vi "OBJ_MAIN.vi"() -> ()   [LabVIEW 2020]
uses:
  OBJ/MAIN/OBJ_header_data_display.ctl
  OBJ/ini/typedef/OBJ_all_config_info.ctl
  OBJ/ini/typedef/OBJ_main_ini_file.ctl
  OBJ/queues/typedef/OBJ_queue_refnums.ctl
  OBJ/queues/typedef/OBJ_MAIN_queue_element.ctl
  OBJ/MAIN/OBJ_MAIN_sequence_state.ctl
  OBJ/queues/typedef/OBJ_SCANNER_queue_element.ctl
  OBJ/SCANNER/OBJ_SCANNER_sequence_state.ctl
  OBJ/queues/typedef/OBJ_MD_queue_element.ctl
  OBJ/MEASURING_DEVICE/OBJ_MD_sequence_state.ctl
  OBJ/queues/typedef/OBJ_GUI_TIMER_queue_element.ctl
  OBJ/GUI_TIMER/OBJ_GUI_TIMER_sequence_state.ctl
  OBJ/FGV/error_buffer/FGV_OBJ_error_buffer.ctl
  OBJ/FGV/SQL_connection/FGV_OBJ_SQL_connection.ctl
  OBJ/FGV/login/FGV_OBJ_login.ctl
  OBJ/FGV/login/OBJ_login_refnums.ctl
  OBJ/FGV/test_button/FGV_OBJ_test_button.ctl
  OBJ/FGV/OBJ_records_display/FGV_OBJ_records_display.ctl
  OBJ/FGV/OBJ_status_display/FGV_OBJ_status_display.ctl
  OBJ/FGV/OBJ_records_display/OBJ_references.ctl
  OBJ/FGV/tristate_indicator_OBJ_test/FGV_tristate_indicator_OBJ_test.ctl
  OBJ/FGV/OBJ_history_display/FGV_OBJ_history_display.ctl
  OBJ/MAIN/OBJ_thread.ctl
  OBJ/FGV/part_number/control_part_number.ctl
  _misc/AULocalize/SubVIs/RegisterVI.vi
  <vilib>/Instr/_visa.llb/VISA Configure Serial Port (Instr).vi
  _misc/AULocalize/SubVIs/Get Localized Phrase Compact Interface 0D.vi
panel:
  out "tooling_name":string caption="Reference:"
  out "app_title":string caption="A603 - OBJ Position"
  in  "professional_timeout_reset_generator":bool
  in  "USER_login_logout":bool
  out "SQL_connections_indicator_global":bool=TRUE caption="SQL Connection Status:"
  out "ERROR_indicator_global":bool caption="Application Status:"
  out "current_access_level":i32=10 caption="Access level:"
  out "current_username":string="jlonga" caption="Logged in as:"
  in  "main_tab":enum32{"OBJ Test", "Errors"}(tab)
  out "input_header":string caption="INPUT"
  in  "OBJ_clear_history":bool
  in  "OBJ_clear_test_data":bool
  out "operator_message":string
  out "test_tristate_indicator":bool
  in  "OBJ_perform_test":bool
  out "OBJ_status":string
  in  "OBJ_gear_serial":string caption="Gear Serial:"
  out "OBJ_header_data_display":T1
  out "gear_info_summary_header":string caption="GEAR INFO SUMMARY"
  out "gear_serial_display":string
  out "OBJ_records":i32(listbox)=-1
  in  "OBJ_history":i32(listbox)=-1
  out "measurement_history_header":string caption="MEASUREMENT HISTORY"
  in  "ERROR_records":i32(listbox)
  in  "ERROR_clear":bool
  out "ERROR_indicator_tab":bool
  in  "STOP":bool
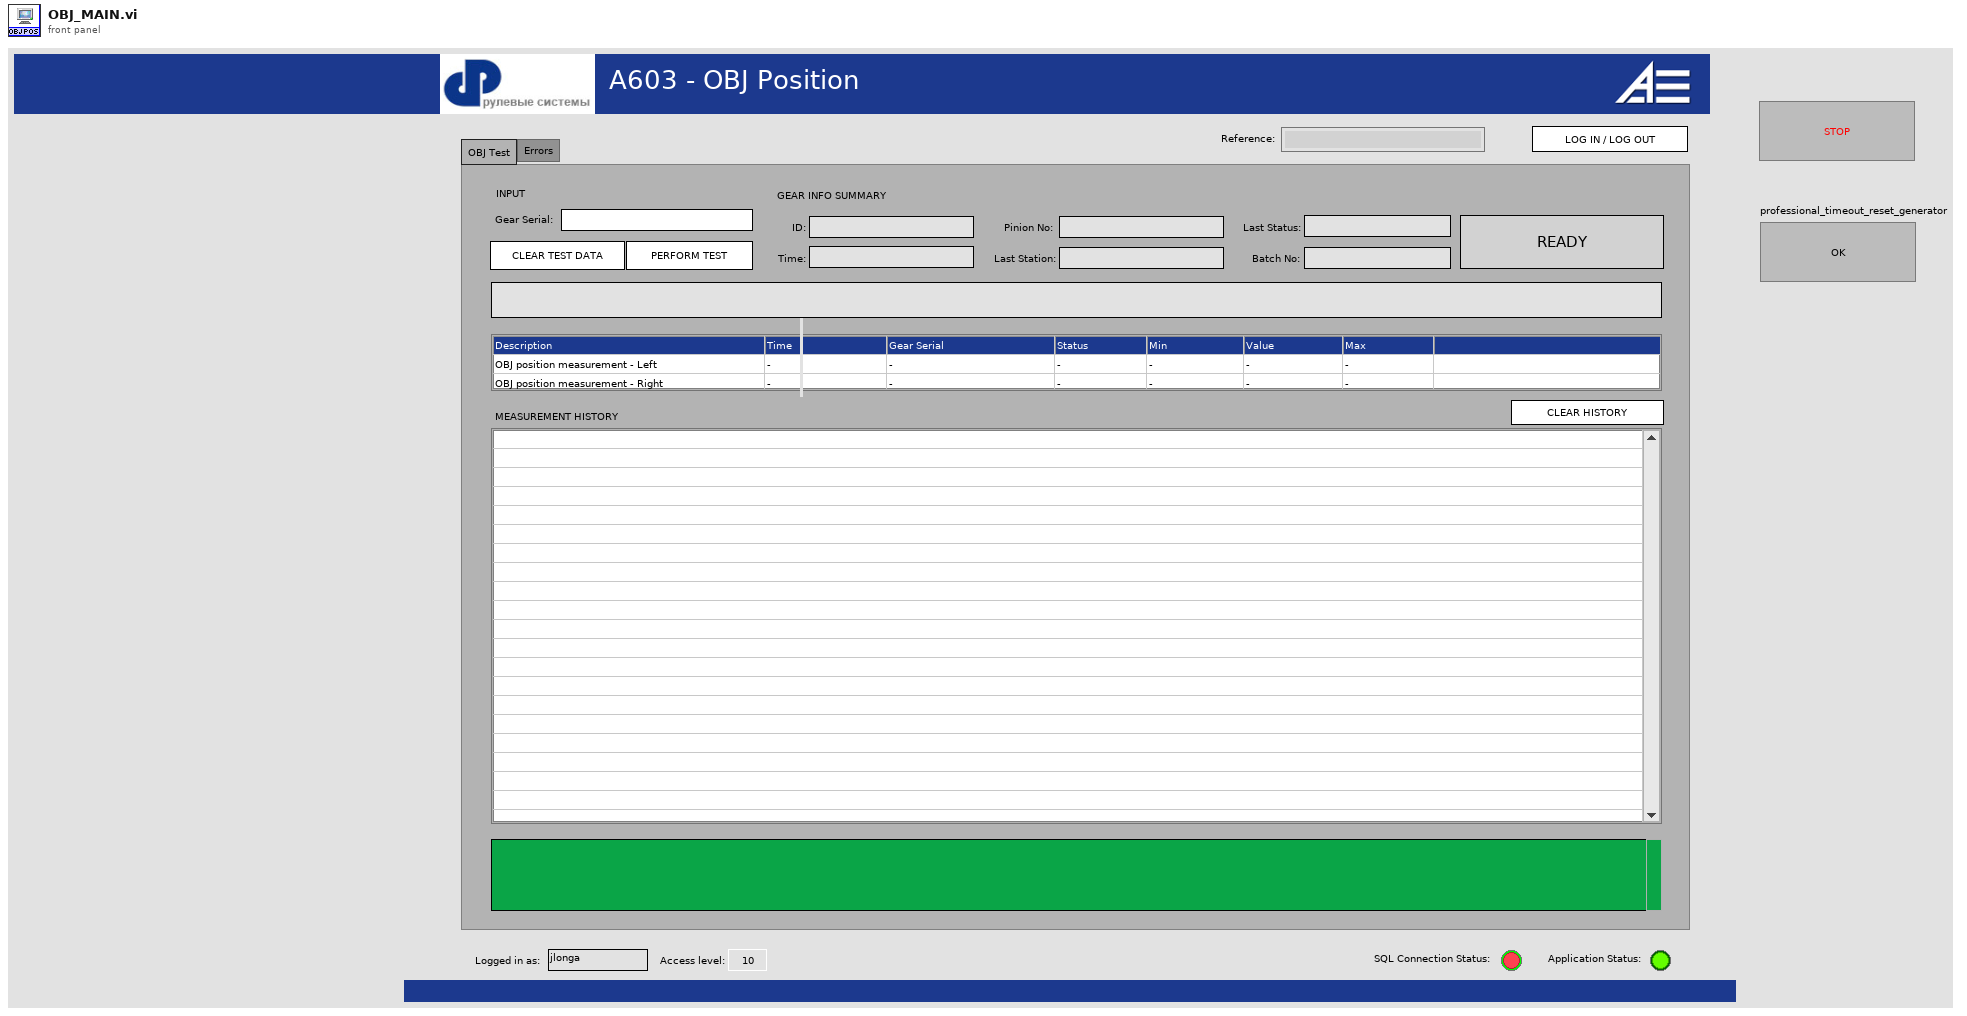
[diagram p1: front panel]
types:
  T1 = typedef "OBJ_header_data_display.ctl" = cluster{"ID":string, "creation_time":string, "last_station":string, "last_status":string, "pinion_serial":string, "batch_code":string}
  T2 = typedef "OBJ_GUI_TIMER_sequence_state.ctl" = enum16{"initialize", "get_next_state", "start_timer", "stop_timer", "timer_finished", "error", "stop"}
  T3 = typedef "FGV_OBJ_history_display.ctl" = enum16{"initialize", "add", "clear"}
  T4 = typedef "OBJ_MD_sequence_state.ctl" = enum16{"initialize", "get_next_state", "get_measurement", "error", "stop"}
  T5 = typedef "FGV_tristate_indicator_OBJ_test.ctl" = enum16{"initialize", "ready", "pending", "OK", "NOK", "part_NOK", "routing_NOK", "repeat_NOK", "timeout", "translate", "error"}
  T6 = typedef "OBJ_references.ctl" = cluster{"front_panel_reference":refnum<vi>, "SQL_listbox_reference":refnum<vi>, "OBJ_header_data_display":refnum<vi>}
  T7 = typedef "FGV_OBJ_status_display.ctl" = enum16{"initialize", "display", "clear"}
  T8 = typedef "FGV_OBJ_records_display.ctl" = enum16{"initialize", "set_serial", "display_header", "display_results", "get_serial", "get_part_ID", "clear"}
  T9 = typedef "OBJ_SCANNER_sequence_state.ctl" = enum16{"initialize", "get_next_state", "read", "error", "stop"}
  T10 = typedef "OBJ_MAIN_sequence_state.ctl" = enum16{"initialize", "get_next_state", "read_reference_list", "USER_login", "USER_logout", "read_gear_data", "perform_test", "start_timer", "clear_test_data", "error", "stop"}
  T11 = typedef "FGV_OBJ_test_button.ctl" = enum16{"initialize", "set_new_login", "set_message", "enable", "disable", "disable_gray", "translate", "set_scan_tooling", "get_scan_tooling"}
  T12 = typedef "OBJ_login_refnums.ctl" = cluster{"current_username":refnum<vi>, "current_access_level":refnum<vi>}
  T13 = typedef "FGV_OBJ_login.ctl" = enum16{"initialize", "start_login_read", "end_login_read", "login", "logout", "get_login_info"}
  T14 = typedef "FGV_OBJ_SQL_connection.ctl" = enum16{"initialize", "connect", "read_tables", "read_columns", "SELECT", "INSERT", "UPDATE", "DELETE", "EXEC + headers", "EXEC", "TRANSACTION", "connection_active?", "disconnect"}
  T15 = typedef "FGV_OBJ_error_buffer.ctl" = enum16{"initialize", "clear", "display", "get_status"}
  T16 = typedef "OBJ_all_config_info.ctl" = cluster{"main_ini_file":T17, "SQL Password":string, "queue_refnums":T18}
  T17 = typedef "OBJ_main_ini_file.ctl" = cluster{"SQL Driver":string, "SQL Server":string, "SQL Database":string, "SQL UID":string, "User table":string, "Reference table":string, "default language":string, "SCANNER COM port":u16, "SCANNER Baud rate":u32, "SCANNER Data bits":u16, "SCANNER Pairity":enum16{"None", "Odd", "Even", "Mark", "Space"}, "SCANNER Stop bits":u16, "SCANNER Flow control":u16, "SCANNER Termination char":u8, "MD-L COM port":u16, "MD-L Baud rate":u32, "MD-L Data bits":u16, "MD-L Pairity":enum16{"None", "Odd", "Even", "Mark", "Space"}, "MD-L Stop bits":u16, "MD-L Flow control":u16, "MD-L Termination char":u8, "MD-R COM port":u16, "MD-R Baud rate":u32, "MD-R Data bits":u16, "MD-R Pairity":enum16{"None", "Odd", "Even", "Mark", "Space"}, "MD-R Stop bits":u16, "MD-R Flow control":u16, "MD-R Termination char":u8, "logout timeout [ms]":i32}
  T18 = typedef "OBJ_queue_refnums.ctl" = cluster{"MAIN_queue":refnum<queue>, "SCANNER_queue":refnum<queue>, "SCANNER_login":refnum<queue>, "MD_L_queue":refnum<queue>, "MD_L_data":refnum<queue>, "MD_R_queue":refnum<queue>, "MD_R_data":refnum<queue>, "OBJ_GUI_TIMER_queue":refnum<queue>}
  T19 = enum8{"Enabled", "Disabled", "Disabled and Grayed Out"}
  T20 = typedef "control_part_number.ctl" = enum16{"set_parts_number", "get_part_number_by_name"}
  T21 = typedef "OBJ_GUI_TIMER_queue_element.ctl" = cluster{"state":T2, "variable":variant}
  T22 = typedef "OBJ_thread.ctl" = enum16{"MAIN", "SCANNER", "MD - LEFT", "MD - RIGHT", "GUI TIMER"}
  T23 = typedef "OBJ_MAIN_queue_element.ctl" = cluster{"state":T10, "variable":variant}
  T24 = typedef "OBJ_SCANNER_queue_element.ctl" = cluster{"state":T9, "variable":variant}
  T25 = typedef "OBJ_MD_queue_element.ctl" = cluster{"state":T4, "variable":variant}
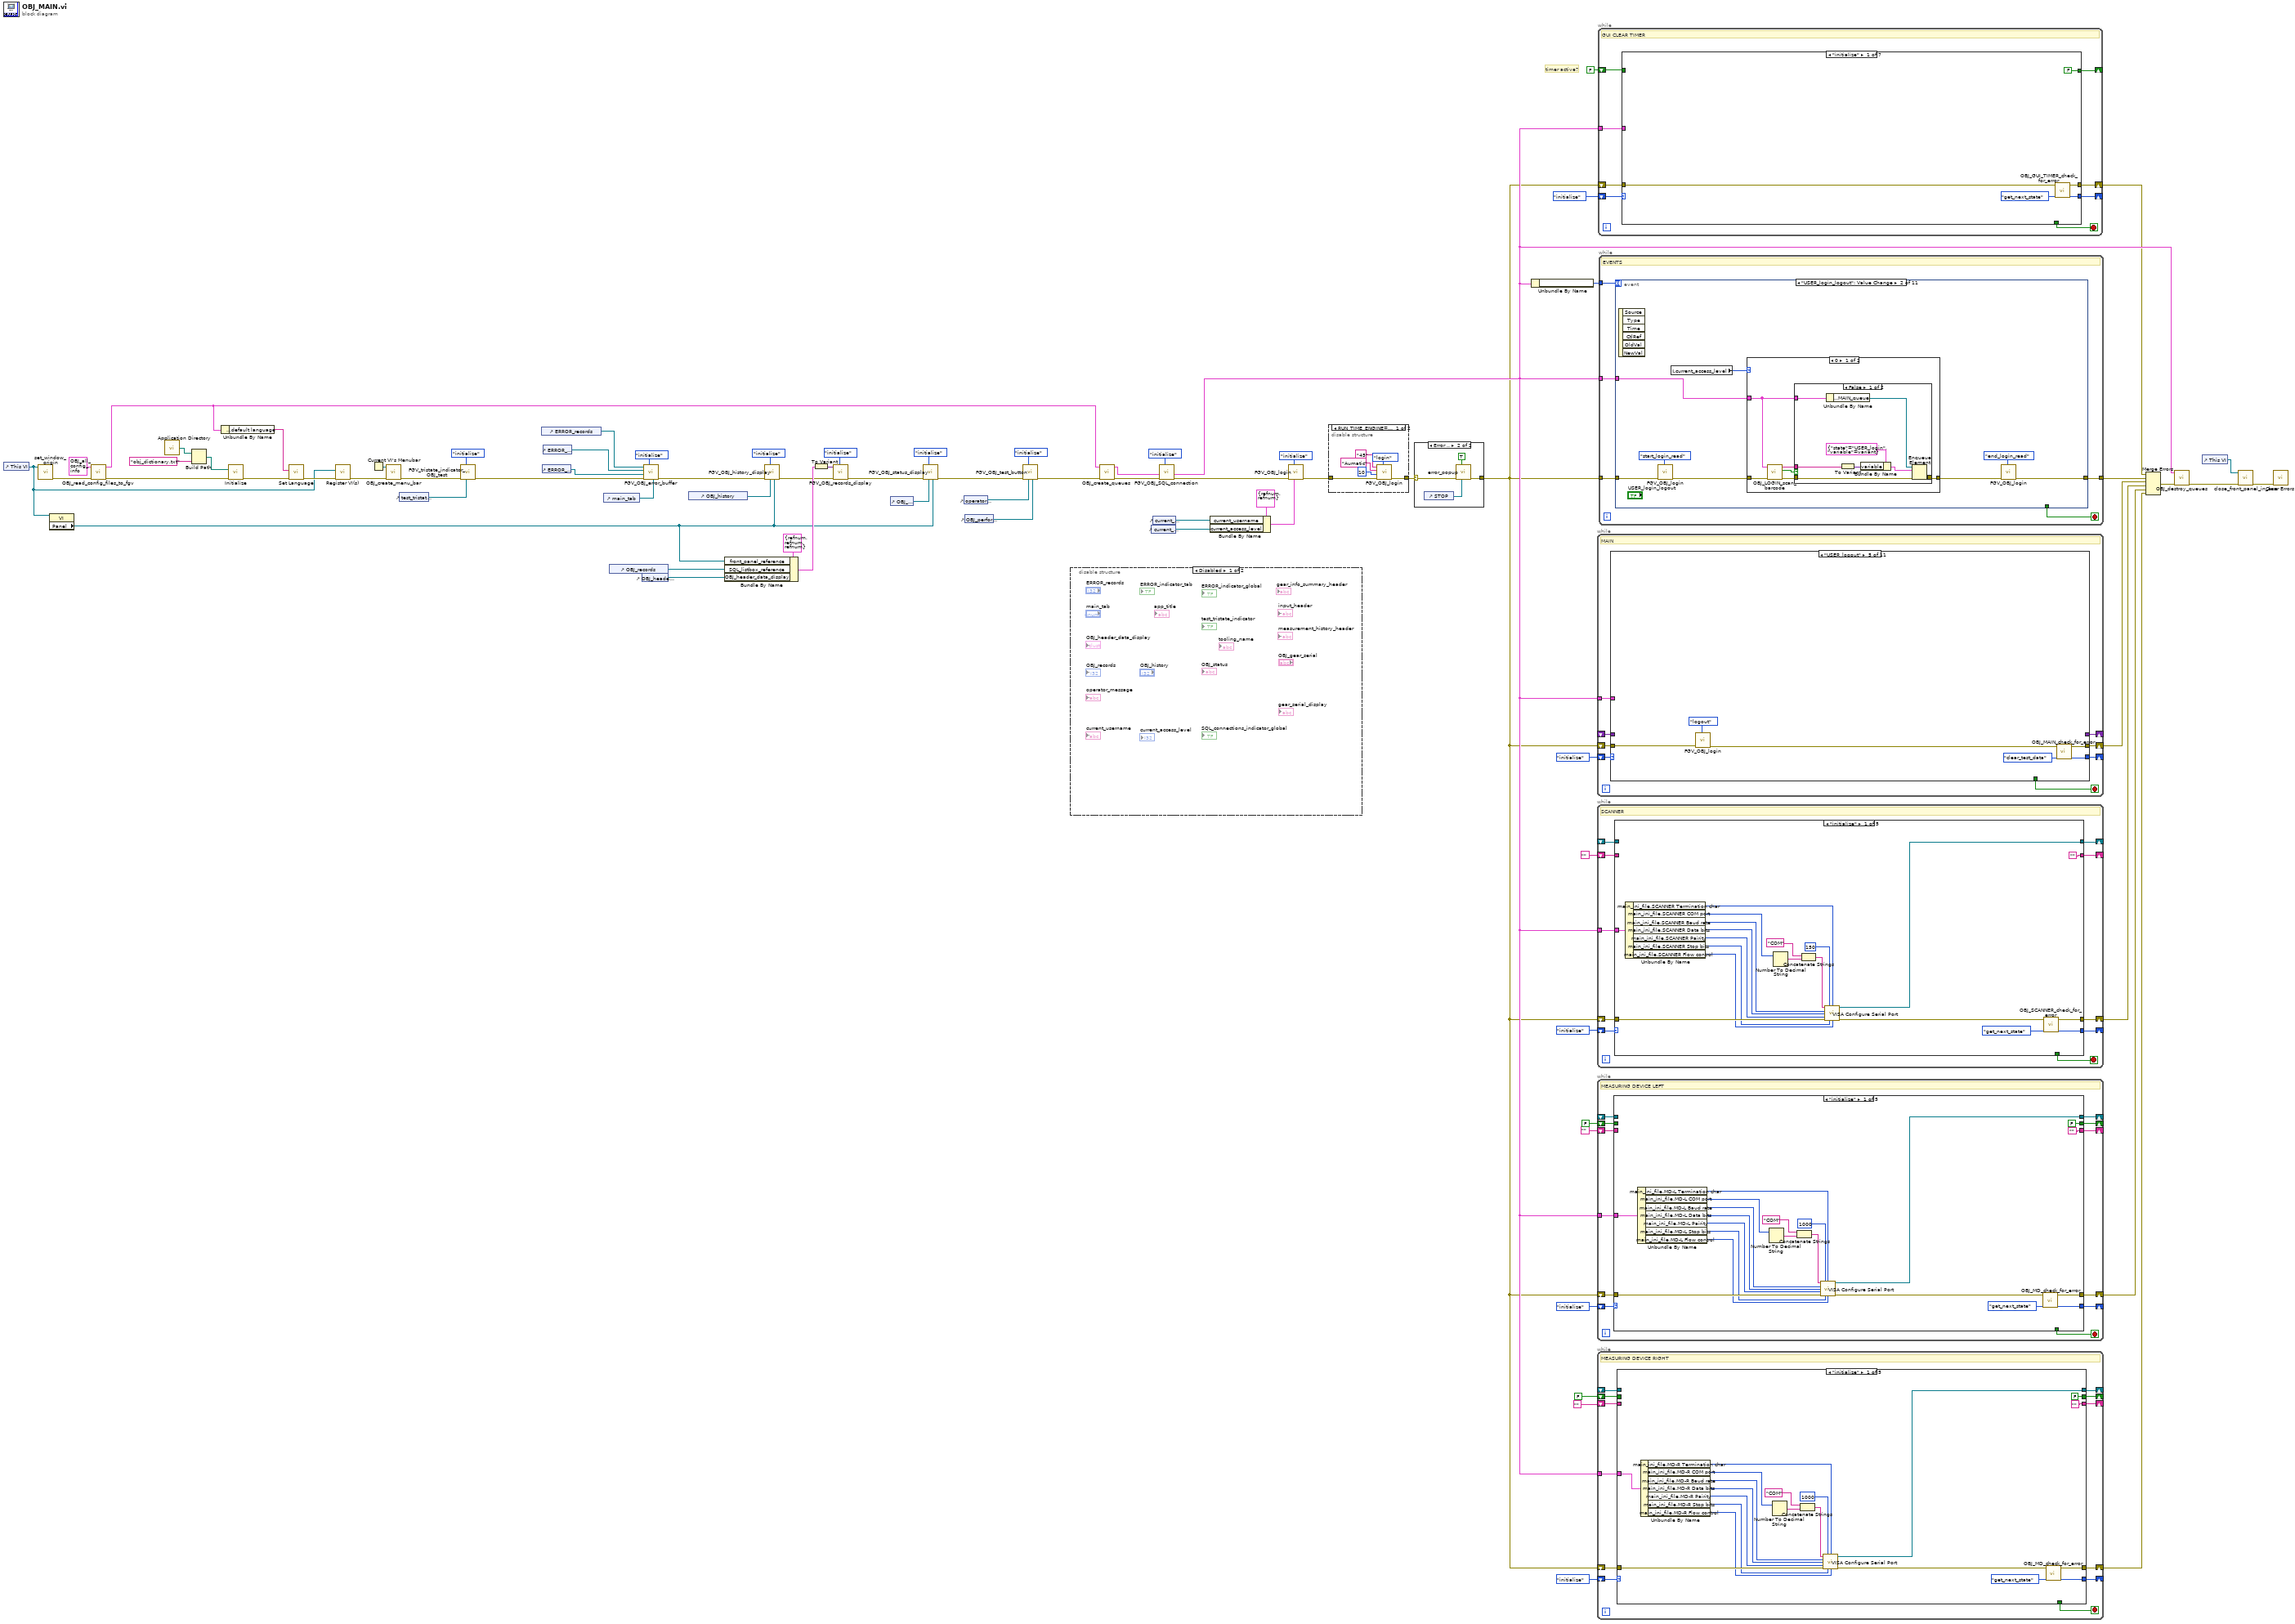
[diagram p0: block diagram]
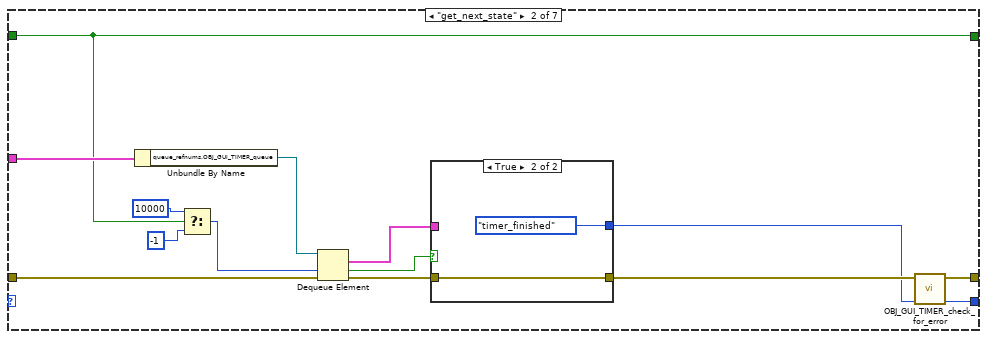
[diagram p3: hidden frame]
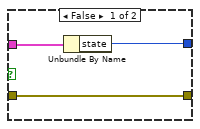
[diagram p4: hidden frame]
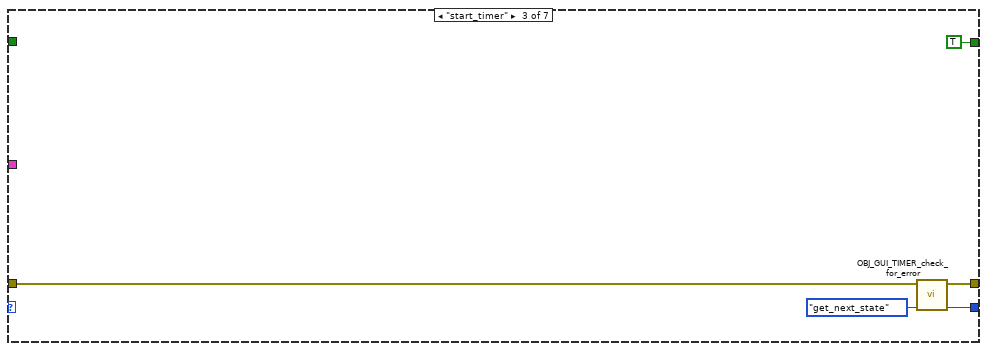
[diagram p5: hidden frame]
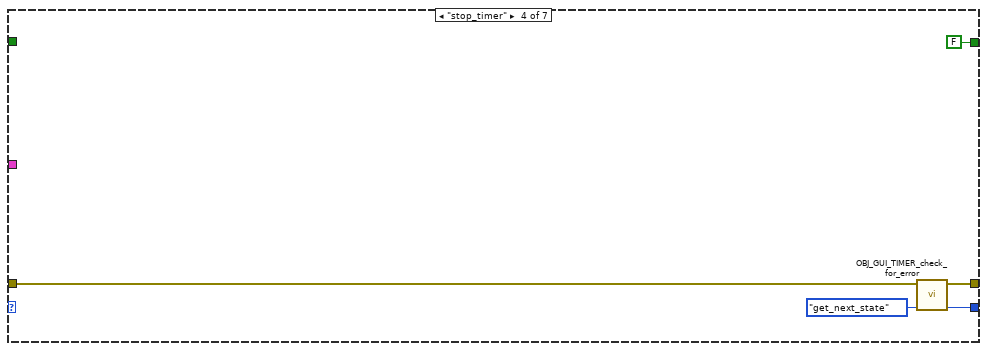
[diagram p6: hidden frame]
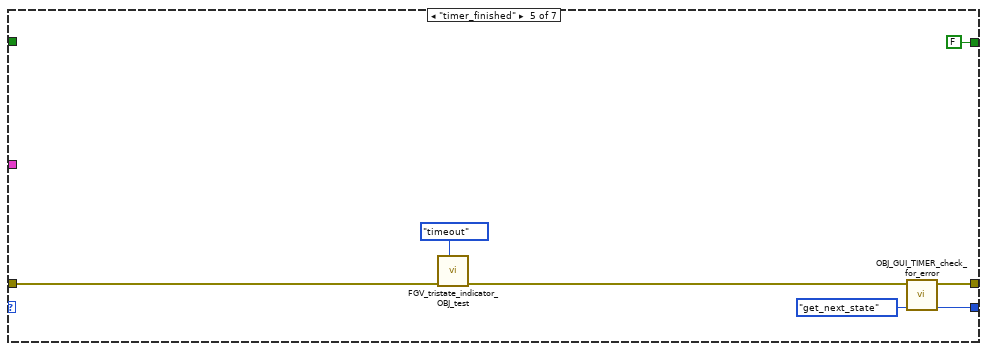
[diagram p7: hidden frame]
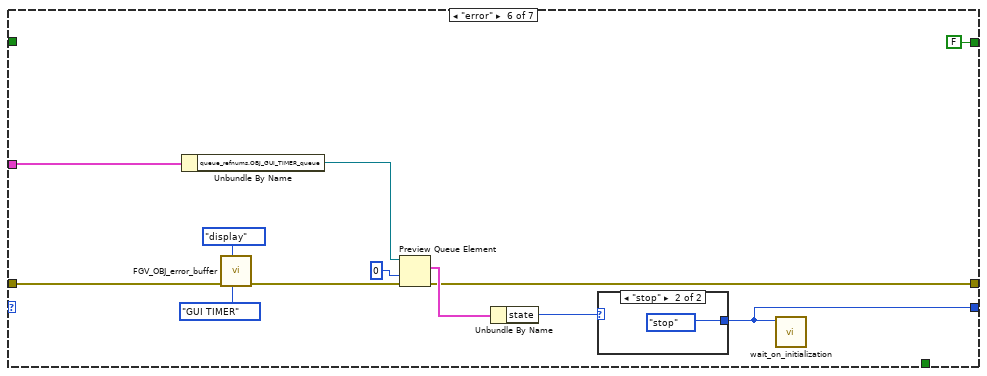
[diagram p8: hidden frame]
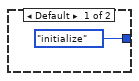
[diagram p9: hidden frame]
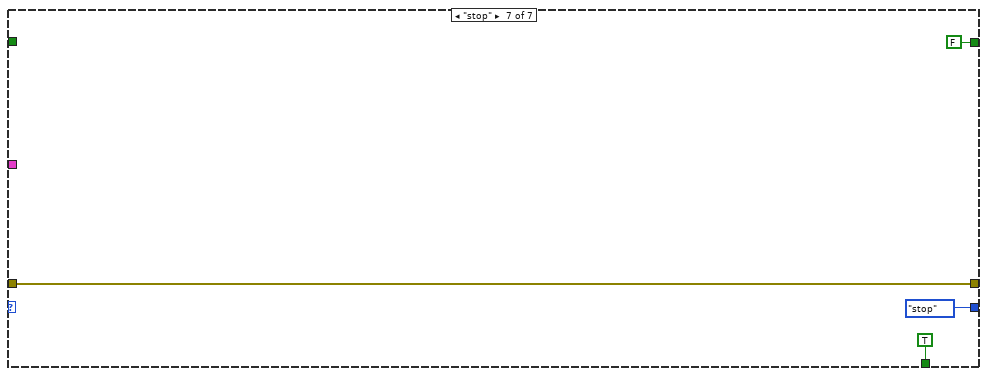
[diagram p10: hidden frame]
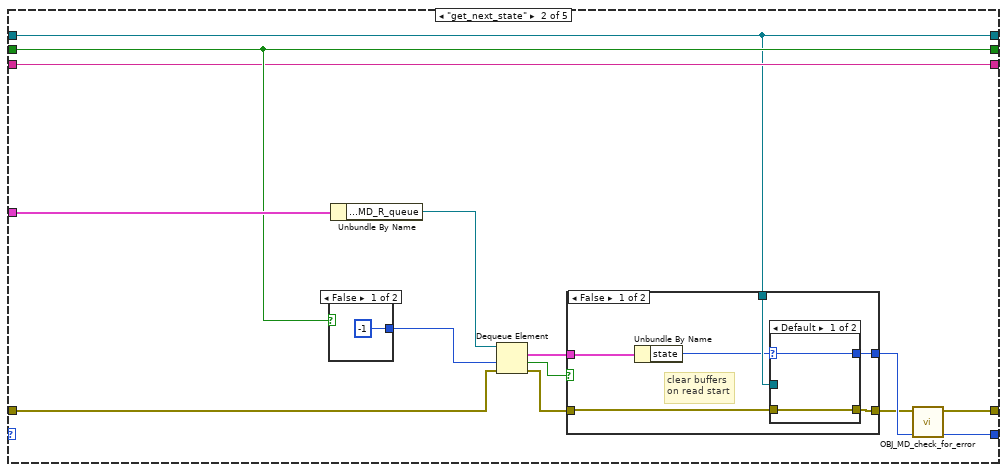
[diagram p12: hidden frame]
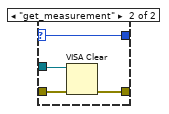
[diagram p13: hidden frame]
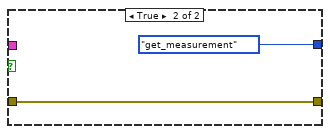
[diagram p14: hidden frame]
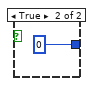
[diagram p15: hidden frame]
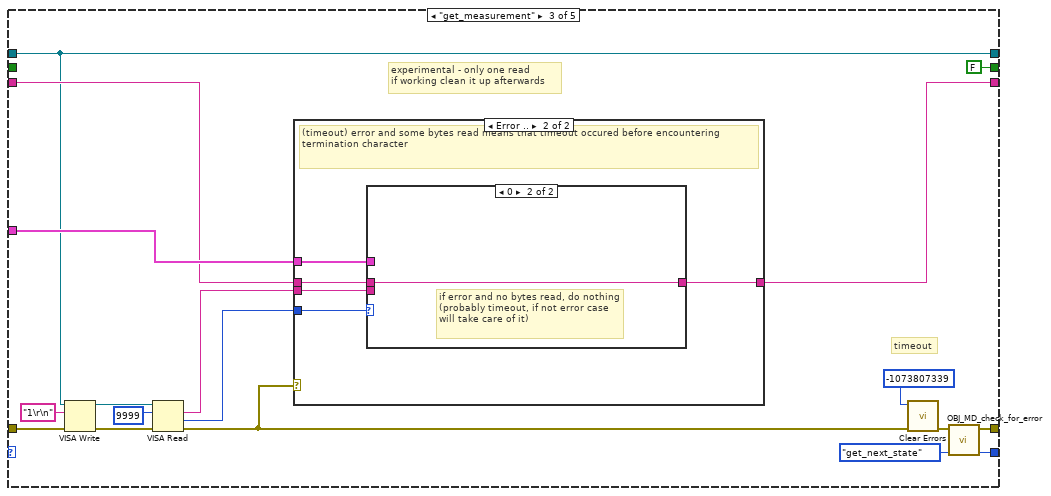
[diagram p16: hidden frame]
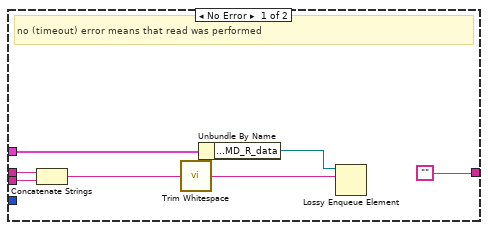
[diagram p17: hidden frame]
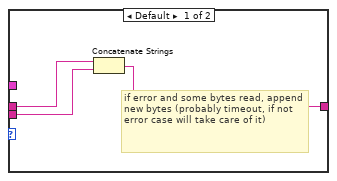
[diagram p18: hidden frame]
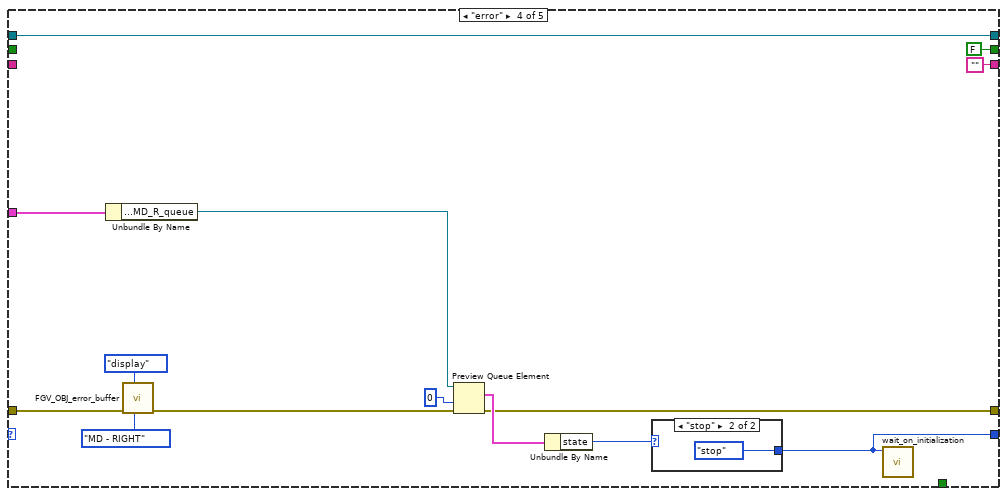
[diagram p19: hidden frame]
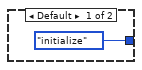
[diagram p20: hidden frame]
diagram:
  # "timer active?"
  n1 = control-ref of="This VI"() -> (w7:refnum<vi>)
  n2 = call "set_window_origin.vi"("this_vi_reference"=w7) -> ("error_out"=w6:errorcluster)  [unwired: 10 in]
  n3 = property class="VI"(reference=w7) -> ("Panel"=w22:refnum<vi>)  [unwired: 1 in, 2 out]
  n4 = call "OBJ_read_config_files_to_fgv.vi"("error_in"=w6, "all_config_info_in"=T16 {"main_ini_file"={"SQL Driver"="", "SQL Server"="", "SQL Database"="", "SQL UID"="", "User table"="", "Reference table"="", "default language"="", "SCANNER COM port"=0, "SCANNER Baud rate"=0, "SCANNER Data bits"=0, "SCANNER Pairity"=enum."None", "SCANNER Stop bits"=10, "SCANNER Flow control"=0, "SCANNER Termination char"=0, "MD-L COM port"=0, "MD-L Baud rate"=0, "MD-L Data bits"=0, "MD-L Pairity"=enum."None", "MD-L Stop bits"=10, "MD-L Flow control"=0, "MD-L Termination char"=0, "MD-R COM port"=0, "MD-R Baud rate"=0, "MD-R Data bits"=0, "MD-R Pairity"=enum."None", "MD-R Stop bits"=10, "MD-R Flow control"=0, "MD-R Termination char"=0, "logout timeout [ms]"=0}, "SQL Password"="", "queue_refnums"={"MAIN_queue"=refnum, "SCANNER_queue"=refnum, "SCANNER_login"=refnum, "MD_L_queue"=refnum, "MD_L_data"=refnum, "MD_R_queue"=refnum, "MD_R_data"=refnum, "OBJ_GUI_TIMER_queue"=refnum}}) -> ("error_out"=w8:errorcluster, "all_config_info_out"=w2:T16)  [unwired: 8 in]
  n5 = call <vilib>:"Application Directory.vi"() -> ("Application Directory"=w13:path)
  n6 = Build Path(base path=w13, name or relative path="obj_dictionary.txt") -> (appended path=w11:path)
  n7 = Unbundle By Name(w2) -> ("main_ini_file.default language"=w1:string)
  n8 = call "Initialize.vi"("Dictionary File Path"=w11, "error in"=w8) -> ("error out"=w10:errorcluster)  [unwired: 8 in, 5 out]
  n9 = call "Set Language.vi"("error in"=w10, "Target Language (current lang)"=w1) -> ("error out"=w9:errorcluster)  [unwired: 8 in, 1 out]
  n10 = call-poly "Register VI(s).vi"("error in"=w9, "VI Ref"=w7) -> ("error out"=w4:errorcluster)  [unwired: 8 in, 1 out]
  n11 = Current VI's Menubar() -> (w5:refnum<k9>)
  n12 = call "OBJ_create_menu_bar.vi"("error_in"=w4, "menu_bar_refnum"=w5) -> ("error_out"=w3:errorcluster)  [unwired: 9 in]
  n13 = control-ref of="test_tristate_indicator"() -> (w33:refnum<vi>)
  n14 = call "FGV_tristate_indicator_OBJ_test.vi"("boolean_indicator_refnum"=w33, "options"=FGV_tristate_indicator_OBJ_test."initialize", "error_in"=w3) -> ("error_out"=w31:errorcluster)  [unwired: 8 in]
  n15 = control-ref of="ERROR_records"() -> (w74:refnum<vi>)
  n16 = control-ref of="ERROR_indicator_global"() -> (w72:refnum<vi>)
  n17 = control-ref of="ERROR_indicator_tab"() -> (w73:refnum<vi>)
  n18 = control-ref of="main_tab"() -> (w26:refnum<vi>)
  n19 = control-ref of="OBJ_records"() -> (w35:refnum<vi>)
  n20 = control-ref of="OBJ_header_data_display"() -> (w20:refnum<vi>)
  n21 = call "FGV_OBJ_error_buffer.vi"("main_tab"=w26, "option"=FGV_OBJ_error_buffer."initialize", "error_in"=w31, "error_indicator_global"=w72, "error_indicator_tab"=w73, "error_display_ref"=w74) -> ("error_out"=w25:errorcluster)  [unwired: 4 in, 1 out]
  n22 = control-ref of="OBJ_history"() -> (w14:refnum<vi>)
  n23 = Bundle By Name(cluster=T6 {"front_panel_reference"=refnum, "SQL_listbox_reference"=refnum, "OBJ_header_data_display"=refnum} ("REWORK_references"), "front_panel_reference"=w22, "SQL_listbox_reference"=w35, "OBJ_header_data_display"=w20) -> (w36:T6)
  n24 = call "FGV_OBJ_history_display.vi"("front_panel_reference"=w22, "history_display_reference"=w14, "options"=FGV_OBJ_history_display."initialize", "error_in"=w25) -> ("error_out"=w24:errorcluster)  [unwired: 7 in]
  n25 = To Variant(anything=w36) -> (Variant=w37:variant)
  n26 = call "FGV_OBJ_records_display.vi"("options"=FGV_OBJ_records_display."initialize", "error_in"=w24, "input"=w37) -> ("error_out"=w43:errorcluster)  [unwired: 7 in, 1 out]
  n27 = control-ref of="OBJ_status"() -> (w39:refnum<vi>)
  n28 = call "FGV_OBJ_status_display.vi"("front_panel_reference"=w22, "status_display_reference"=w39, "options"=FGV_OBJ_status_display."initialize", "error_in"=w43) -> ("error_out"=w42:errorcluster)  [unwired: 7 in]
  n29 = control-ref of="operator_message"() -> (w51:refnum<vi>)
  n30 = control-ref of="OBJ_perform_test"() -> (w52:refnum<vi>)
  n31 = call "FGV_OBJ_test_button.vi"("OBJ_test_button"=w52, "operator_message"=w51, "options"=FGV_OBJ_test_button."initialize", "error_in"=w42) -> ("error_out"=w32:errorcluster)  [unwired: 6 in, 1 out]
  n32 = disable-structure shown="Disabled" {
    frame Disabled {
    }
    frame Enabled {
    }
  }
  n33 = call "OBJ_create_queues.vi"("error_in"=w32, "all_config_info_in"=w2) -> ("error_out"=w62:errorcluster, "all_config_info_out"=w60:T16)  [unwired: 8 in]
  n34 = control-ref of="current_access_level"() -> (w54:refnum<vi>)
  n35 = control-ref of="current_username"() -> (w55:refnum<vi>)
  n36 = call "FGV_OBJ_SQL_connection.vi"("options"=FGV_OBJ_SQL_connection."initialize", "error_in"=w62, "all_config_info_in"=w60) -> ("error_out"=w59:errorcluster, "all_config_info_out"=w19:T16)  [unwired: 4 in, 3 out]
  n37 = Bundle By Name(cluster=T12 {"current_username"=refnum, "current_access_level"=refnum} ("login_refnums"), "current_username"=w55, "current_access_level"=w54) -> (w56:T12)
  n38 = call "FGV_OBJ_login.vi"("login_refnums"=w56, "options"=FGV_OBJ_login."initialize", "error_in"=w59) -> ("error_out"=w53:errorcluster)  [unwired: 4 in, 4 out]
  n39 = disable-structure shown="RUN_TIME_ENGINE==False" {
    disable-tunnel: w53 -> [w82 w83]
    disable-tunnel: [w81 w83] -> w30
    frame condition #0 (active) {
      n40 = call "FGV_OBJ_login.vi"("options"=FGV_OBJ_login."login", "error_in"=w82, "access_level_in"=10, "username_in"="Aumatic", "ID_in"="45") -> ("error_out"=w81:errorcluster)  [unwired: 2 in, 4 out]
    }
    frame condition #1 {
    }
  }
  n41 = case shown="Error .." w30 {
    selector: w30 -> [w84 w87]
    tunnel: [w84 w88] -> w17
    frame No Error {
    }
    frame Error {
      n42 = control-ref of="STOP"() -> (w86:refnum<vi>)
      n43 = call "error_popup.vi"("STOP_button_reference"=w86, "EXIT App If Error? (F)"=TRUE, "error_in"=w87) -> ("error_out"=w88:errorcluster)  [unwired: 8 in]
    }
  }
  n44 = Unbundle By Name(w19) -> ("main_ini_file.logout timeout [ms]"=w21:i32)
  n45 = while {
    tunnel: w19 -> [w92]
    shift-right: [w93] -> _
    shift-left: OBJ_MAIN_sequence_state."initialize" ("state") -> [w94]
    shift-right: [w91] -> _
    shift-left: _ -> [w90]
    shift-right: [w95] -> w66
    shift-left: w17 -> [w96]
    stop <- w89 stop-if-true
    # "MAIN"
    n46 = case shown="\"USER_logout\"" w94 {
      tunnel: w96 -> [w101 w109 w120 w138 w181 w213 w226 w272 w288 w296 w320]
      tunnel: [w104 w113 w132 w137 w177 w208 w223 w276 w279 w298 w320] -> w95
      tunnel: [w102 w112 w131 w134 w178 w207 w222 w275 w278 w297 OBJ_MAIN_sequence_state."stop" ("ST_TCP_sequence_state")] -> w93
      tunnel: w92 -> [_ w107 w118 w136 _ _ w232 w273 _ w292 _]
      tunnel: [_ w105 _ _ _ _ _ _ _ _ _] -> w91
      tunnel: w90 -> [_ _ _ w135 _ w214 _ _ _ _ _]
      tunnel: [_ _ _ _ _ _ _ _ _ _ TRUE] -> w89
      frame "initialize" {
        n47 = call "FGV_OBJ_SQL_connection.vi"("options"=FGV_OBJ_SQL_connection."connect", "error_in"=w101) -> ("error_out"=w98:errorcluster)  [unwired: 5 in, 4 out]
        n48 = Unbundle By Name(w98) -> ("status"=w97:bool)
        n49 = local write "SQL_connections_indicator_global"(w97) -> ()
        n50 = local write "gear_serial_display"("") -> ()
        n51 = call "OBJ_MAIN_check_for_error.vi"("MAIN_loop_state_in"=OBJ_MAIN_sequence_state."get_next_state", "error_in"=w98) -> ("MAIN_loop_state_out"=w102:T10, "error_out"=w104:errorcluster)  [unwired: 8 in]
      }
      frame "get_next_state" {
        n52 = Unbundle By Name(w107) -> ("queue_refnums.MAIN_queue"=w110:refnum<queue>)
        n53 = Dequeue Element(queue=w110, error in (no error)=w109) -> (element=w111:T23, error out=w108:errorcluster)  [unwired: 1 in, 2 out]
        n54 = Unbundle By Name(w111) -> ("variable"=w105:variant, "state"=w106:T10)
        n55 = call "OBJ_MAIN_check_for_error.vi"("MAIN_loop_state_in"=w106, "error_in"=w108) -> ("MAIN_loop_state_out"=w112:T10, "error_out"=w113:errorcluster)  [unwired: 8 in]
      }
      frame "read_reference_list" {
        n56 = Unbundle By Name(w118) -> ("main_ini_file.Reference table"=w125:string)
        n57 = Format Into String(format string="SELECT REFERENCE_NAME, VALUE FROM %s WHERE DESCRIPTION = 'Part number' AND STATION_NMB = 160", w125) -> (resulting string=w126:string)  [unwired: 2 in, 1 out]
        n58 = call "FGV_OBJ_SQL_connection.vi"("options"=FGV_OBJ_SQL_connection."EXEC", "error_in"=w120, "SQL_statement"=w126) -> ("error_out"=w128:errorcluster, "SQL_result"=w130:variant, "executed_SQL_statement"=w127:string)  [unwired: 4 in, 2 out]
        n59 = Variant To Data(error in=w128, type=string[][] [], Variant=w130) -> (data=w116:string[][], error out=w129:errorcluster)
        n60 = property on="tooling_name" class="Str"("DisabledEnum"=T19."Disabled" ("Disabled")) -> ()  [unwired: 2 in, 2 out]
        n61 = call "control_part_number.vi"("select_for_part_number"=control_part_number."set_parts_number", "parts_number"=w116) -> ()  [unwired: 8 in, 2 out]
        n62 = call "FGV_OBJ_status_display.vi"("options"=FGV_OBJ_status_display."display", "error_in"=w129, "SQL_statement"=w127, "display_source"="READ REFERENCE LIST") -> ("error_out"=w119:errorcluster)  [unwired: 7 in]
        n63 = call "OBJ_MAIN_check_for_error.vi"("error_in"=w119) -> ("MAIN_loop_state_out"=w131:T10, "error_out"=w132:errorcluster)  [unwired: 9 in]
      }
      frame "USER_login" {
        n64 = Variant To Data(error in=w138, type="", Variant=w135) -> (data=w144:string, error out=w153:errorcluster)
        n65 = Unbundle By Name(w136) -> ("main_ini_file.User table"=w149:string)
        n66 = call "Hash String with SHA-256.vi"("error_n"=w153, "string"=w144) -> ("error_out"=w150:errorcluster, "hash"=w143:string)  [unwired: 8 in]
        n67 = Format Into String(format string="select ID, USER_NAME, PROXY_APP\nfrom %s\nwhere BARCODE_HASH = '%s'\norder by ID desc", w149, w143) -> (resulting string=w152:string)  [unwired: 2 in, 1 out]
        n68 = call "FGV_OBJ_SQL_connection.vi"("options"=FGV_OBJ_SQL_connection."SELECT", "error_in"=w150, "SQL_statement"=w152) -> ("error_out"=w151:errorcluster, "SQL_result"=w148:variant)  [unwired: 4 in, 3 out]
        n69 = Variant To Data(error in=w151, type=string[][] [], Variant=w148) -> (data=w146:string[][], error out=w147:errorcluster)
        n70 = Empty Array?(array=w146) -> (empty?=w145:bool)
        n71 = case shown="True" w145 {
          tunnel: [w165 w173] -> w154
          tunnel: w147 -> [w163 w174]
          tunnel: w146 -> [w160 _]
          tunnel: w144 -> [_ w169]
          tunnel: w143 -> [_ w168]
          frame False {
            w158 = 0 ("index (row)")
            n72 = Index Array(array=w160, index (row) #2=w158, index (col) #2=w158, index (row) #3=w158, index (col) #3=1 ("disabled index (col)"), index (row) #4=w158, index (col) #4=2 ("disabled index (col)")) -> (element #2=w162:string, element #3=w155:string, element #4=w156:string)  [unwired: 2 in, 1 out]
            n73 = Decimal String To Number(string=w156) -> (number=w159:i32)  [unwired: 2 in, 1 out]
            n74 = call "FGV_OBJ_login.vi"("options"=FGV_OBJ_login."login", "error_in"=w163, "access_level_in"=w159, "username_in"=w155, "ID_in"=w162) -> ("error_out"=w165:errorcluster)  [unwired: 2 in, 4 out]
          }
          frame True {
            n75 = call-poly "Get Localized Phrase Compact Interface.vi"("Key"="Scanned card not in database!\nCard: %s\nHash: %s" ("Message")) -> ("Translated Phrase"=w166:string)
            n76 = Format Into String(format string=w166, w169, w168) -> (resulting string=w167:string)  [unwired: 2 in, 1 out]
            n77 = call "message_popup.vi"("Warning(T)/Info(F)"=TRUE, "error_in"=w174, "Message"=w167, "Title"="Login", "Button Label"="OK") -> ("error_out"=w173:errorcluster)  [unwired: 6 in]
          }
        }
        n78 = call "OBJ_MAIN_check_for_error.vi"("MAIN_loop_state_in"=OBJ_MAIN_sequence_state."get_next_state", "error_in"=w154) -> ("MAIN_loop_state_out"=w134:T10, "error_out"=w137:errorcluster)  [unwired: 8 in]
      }
      frame "USER_logout" {
        n79 = call "FGV_OBJ_login.vi"("options"=FGV_OBJ_login."logout", "error_in"=w181) -> ("error_out"=w176:errorcluster)  [unwired: 5 in, 4 out]
        n80 = call "OBJ_MAIN_check_for_error.vi"("MAIN_loop_state_in"=OBJ_MAIN_sequence_state."clear_test_data", "error_in"=w176) -> ("MAIN_loop_state_out"=w178:T10, "error_out"=w177:errorcluster)  [unwired: 8 in]
      }
      frame "read_gear_data" {
        n81 = Variant To Data(error in=w213, type="", Variant=w214) -> (data=w182:string, error out=w185:errorcluster)
        n82 = call "FGV_OBJ_records_display.vi"("options"=FGV_OBJ_records_display."clear", "error_in"=w185) -> ("error_out"=w183:errorcluster)  [unwired: 8 in, 1 out]
        n83 = To Variant(anything="READING GEAR DATA" ("data")) -> (Variant=w197:variant)
        n84 = call "FGV_OBJ_test_button.vi"("options"=FGV_OBJ_test_button."set_message", "error_in"=w183, "input"=w197) -> ("error_out"=w194:errorcluster)  [unwired: 7 in, 1 out]
        n85 = To Variant(anything=w182) -> (Variant=w200:variant)
        n86 = call "FGV_OBJ_records_display.vi"("options"=FGV_OBJ_records_display."set_serial", "error_in"=w183, "input"=w200) -> ()  [unwired: 7 in, 2 out]
        n87 = call "FGV_tristate_indicator_OBJ_test.vi"("options"=FGV_tristate_indicator_OBJ_test."pending", "error_in"=w194) -> ("error_out"=w193:errorcluster)  [unwired: 9 in]
        n88 = local write "OBJ_gear_serial"(w182) -> ()
        n89 = local write "gear_serial_display"(w182) -> ()
        n90 = Format Into String(format string="EXEC CheckIfOperationValidOBJ @PartSerial = '%s'" ("SQL_statement"), w182) -> (resulting string=w209:string)  [unwired: 2 in, 1 out]
        n91 = call "FGV_OBJ_SQL_connection.vi"("options"=FGV_OBJ_SQL_connection."EXEC", "error_in"=w193, "SQL_statement"=w209) -> ("error_out"=w202:errorcluster, "SQL_result"=w190:variant, "executed_SQL_statement"=w205:string)  [unwired: 4 in, 2 out]
        n92 = call "FGV_OBJ_records_display.vi"("options"=FGV_OBJ_records_display."display_header", "error_in"=w202, "input"=w190) -> ("error_out"=w192:errorcluster)  [unwired: 7 in, 1 out]
        n93 = call "OBJ_parse_read_gear_data_response.vi"("error_in"=w192, "recordset_in"=w190) -> ("error_out"=w191:errorcluster, "Perform test?"=w189:bool)  [unwired: 8 in]
        n94 = Select(t=OBJ_MAIN_sequence_state."perform_test", s=w189, f=OBJ_MAIN_sequence_state."get_next_state" ("ST_TCP_sequence_state")) -> (s? t:f=w187:T10)
        n95 = call "FGV_OBJ_status_display.vi"("options"=FGV_OBJ_status_display."display", "error_in"=w191, "SQL_statement"=w205, "display_source"="GEAR DATA READ") -> ("error_out"=w206:errorcluster)  [unwired: 7 in]
        n96 = call "OBJ_MAIN_check_for_error.vi"("MAIN_loop_state_in"=w187, "error_in"=w206) -> ("MAIN_loop_state_out"=w207:T10, "error_out"=w208:errorcluster)  [unwired: 8 in]
      }
      frame "perform_test" {
        n97 = To Variant(anything="READING MEASUREMENTS" ("data")) -> (Variant=w228:variant)
        n98 = property on="professional_timeout_reset_generator" class="Bool (strict)"("Val(Sgnl)"=TRUE ("Value (Signaling)")) -> ()  [unwired: 2 in, 2 out]
        n99 = call "FGV_OBJ_test_button.vi"("options"=FGV_OBJ_test_button."set_message", "error_in"=w226, "input"=w228) -> ("error_out"=w225:errorcluster)  [unwired: 7 in, 1 out]
        n100 = call "OBJ_MAIN_get_test_data.vi"("error_in"=w225, "all_config_info"=w232) -> ("error_out"=w231:errorcluster, "Timed out?"=w215:bool, "measurement_right"=w230:string, "measurement_left"=w216:string)  [unwired: 6 in]
        n101 = case shown="False" w215 {
          tunnel: w231 -> [w243 w264]
          tunnel: [w236 w262] -> w224
          tunnel: w216 -> [w246 _]
          tunnel: w230 -> [w245 _]
          tunnel: [w234 FALSE ("test_ok?")] -> w221
          frame False {
            # "READING OK"
            n102 = To Variant(anything="SAVING RESULTS" ("data")) -> (Variant=w244:variant)
            n103 = call "FGV_OBJ_test_button.vi"("options"=FGV_OBJ_test_button."set_message", "error_in"=w243, "input"=w244) -> ("error_out"=w242:errorcluster)  [unwired: 7 in, 1 out]
            n104 = call "FGV_OBJ_records_display.vi"("options"=FGV_OBJ_records_display."get_part_ID", "error_in"=w242) -> ("error_out"=w256:errorcluster, "output"=w255:variant)  [unwired: 8 in]
            n105 = Variant To Data(error in=w256, type="", Variant=w255) -> (data=w253:string, error out=w252:errorcluster)
            n106 = call "FGV_OBJ_login.vi"("options"=FGV_OBJ_login."get_login_info", "error_in"=w252) -> ("error_out"=w249:errorcluster, "ID_out"=w250:string)  [unwired: 5 in, 3 out]
            n107 = Format Into String(format string="EXEC SaveResultsOBJ @ReferenceName = '%s', @MeasurementLeft = '%s', @MeasurementRight = '%s', @PartID = '%s', @UserID = '%s'" ("SQL_statement"), "", w246, w245, w253, w250) -> (resulting string=w259:string)  [unwired: 2 in, 1 out]
            n108 = call "FGV_OBJ_SQL_connection.vi"("options"=FGV_OBJ_SQL_connection."EXEC", "error_in"=w249, "SQL_statement"=w259) -> ("error_out"=w248:errorcluster, "SQL_result"=w247:variant, "executed_SQL_statement"=w235:string)  [unwired: 4 in, 2 out]
            n109 = call "OBJ_parse_result_save_response.vi"("error_in"=w248, "measurement_right"=w245, "measurement_left"=w246, "sql_results_in"=w247) -> ("error_out"=w237:errorcluster, "test_ok?"=w234:bool)  [unwired: 6 in]
            n110 = call "FGV_OBJ_status_display.vi"("options"=FGV_OBJ_status_display."display", "error_in"=w237, "SQL_statement"=w235, "display_source"="RESULTS SAVE") -> ("error_out"=w236:errorcluster)  [unwired: 7 in]
          }
          frame True {
            # "READING TIMED OUT"
            n111 = call "FGV_tristate_indicator_OBJ_test.vi"("options"=FGV_tristate_indicator_OBJ_test."NOK", "error_in"=w264) -> ("error_out"=w263:errorcluster)  [unwired: 9 in]
            n112 = To Variant(anything="DEVICE READ TIMED OUT - CHECK ERRORS") -> (Variant=w266:variant)
            n113 = call "FGV_OBJ_test_button.vi"("options"=FGV_OBJ_test_button."set_message", "error_in"=w263, "input"=w266) -> ("error_out"=w262:errorcluster)  [unwired: 7 in, 1 out]
          }
        }
        n114 = Select(t=OBJ_MAIN_sequence_state."start_timer", s=w221, f=OBJ_MAIN_sequence_state."get_next_state" ("ST_TCP_sequence_state")) -> (s? t:f=w218:T10)
        n115 = call "OBJ_MAIN_check_for_error.vi"("MAIN_loop_state_in"=w218, "error_in"=w224) -> ("MAIN_loop_state_out"=w222:T10, "error_out"=w223:errorcluster)  [unwired: 8 in]
      }
      frame "start_timer" {
        n116 = Unbundle By Name(w273) -> ("queue_refnums.OBJ_GUI_TIMER_queue"=w271:refnum<queue>)
        n117 = Enqueue Element(queue=w271, element=T21 {"state"=enum."start_timer", "variable"=variant}, error in (no error)=w272) -> (error out=w270:errorcluster)  [unwired: 1 in, 2 out]
        n118 = call "OBJ_MAIN_check_for_error.vi"("MAIN_loop_state_in"=OBJ_MAIN_sequence_state."get_next_state", "error_in"=w270) -> ("MAIN_loop_state_out"=w275:T10, "error_out"=w276:errorcluster)  [unwired: 8 in]
      }
      frame "clear_test_data" {
        n119 = call "FGV_OBJ_records_display.vi"("options"=FGV_OBJ_records_display."clear", "error_in"=w288) -> ("error_out"=w277:errorcluster)  [unwired: 8 in, 1 out]
        n120 = call "FGV_OBJ_status_display.vi"("options"=FGV_OBJ_status_display."clear", "error_in"=w277) -> ("error_out"=w282:errorcluster)  [unwired: 9 in]
        n121 = local write "gear_serial_display"("") -> ()
        n122 = To Variant(anything="READY FOR TEST") -> (Variant=w286:variant)
        n123 = call "FGV_OBJ_test_button.vi"("options"=FGV_OBJ_test_button."set_message", "error_in"=w282, "input"=w286) -> ("error_out"=w283:errorcluster)  [unwired: 7 in, 1 out]
        n124 = call "FGV_tristate_indicator_OBJ_test.vi"("options"=FGV_tristate_indicator_OBJ_test."ready", "error_in"=w283) -> ("error_out"=w280:errorcluster)  [unwired: 9 in]
        n125 = call "OBJ_MAIN_check_for_error.vi"("MAIN_loop_state_in"=OBJ_MAIN_sequence_state."get_next_state", "error_in"=w280) -> ("MAIN_loop_state_out"=w278:T10, "error_out"=w279:errorcluster)  [unwired: 8 in]
      }
      frame "error" {
        n126 = call "FGV_OBJ_error_buffer.vi"("thread"=OBJ_thread."MAIN", "option"=FGV_OBJ_error_buffer."display", "error_in"=w296) -> ("error_out"=w295:errorcluster)  [unwired: 7 in, 1 out]
        n127 = call "FGV_OBJ_SQL_connection.vi"("options"=FGV_OBJ_SQL_connection."connection_active?", "error_in"=w295) -> ("error_out"=w301:errorcluster, "connection_active?"=w300:bool)  [unwired: 5 in, 3 out]
        n128 = case shown="False" w300 {
          tunnel: [w307 OBJ_MAIN_sequence_state."get_next_state" ("ST_TCP_sequence_state")] -> w297
          tunnel: [w305 w316] -> w298
          tunnel: w301 -> [w310 w316]
          tunnel: w292 -> [w303 _]
          frame False {
            # "ERROR WITH CONNECTION"
            n129 = Unbundle By Name(w303) -> ("queue_refnums.MAIN_queue"=w302:refnum<queue>)
            n130 = local write "SQL_connections_indicator_global"(TRUE ("SQL_connections_indicator_global")) -> ()
            n131 = call "FGV_OBJ_SQL_connection.vi"("options"=FGV_OBJ_SQL_connection."disconnect", "error_in"=w310) -> ("error_out"=w313:errorcluster)  [unwired: 5 in, 4 out]
            n132 = call <vilib>:"Clear Errors.vi"("error in (no error)"=w313) -> ("error out"=w306:errorcluster)  [unwired: 5 in, 1 out]
            n133 = Preview Queue Element(queue=w302, timeout in ms (-1)=0, error in (no error)=w306) -> (element=w309:T23, error out=w305:errorcluster)  [unwired: 2 out]
            n134 = Unbundle By Name(w309) -> ("state"=w304:T10)
            n135 = case shown="\"stop\"" w304 {
              tunnel: [OBJ_MAIN_sequence_state."initialize" ("ST_TCP_sequence_state") OBJ_MAIN_sequence_state."stop" ("ST_TCP_sequence_state")] -> w307
              frame Default {
              }
              frame "stop" {
              }
            }
          }
          frame True {
            # "ERROR WITH SQL STATEMENT OR SIMILAR"
          }
        }
        n136 = call "wait_on_initialization.vi"("state"=w297) -> ()  [unwired: 11 in]
      }
      frame "stop" {
      }
    }
  }
  n137 = while {
    tunnel: w19 -> [w327]
    shift-right: [w326] -> _
    shift-left: OBJ_SCANNER_sequence_state."initialize" ("REWORK_SCANNER_sequence_state") -> [w321]
    shift-right: [w324] -> _
    shift-left: "" -> [w322]
    shift-right: [w325] -> _
    shift-left: _ -> [w323]
    shift-right: [w329] -> w65
    shift-left: w17 -> [w330]
    stop <- w328 stop-if-true
    # "SCANNER"
    n138 = case shown="\"initialize\"" w321 {
      tunnel: w330 -> [w346 w361 w378 w424 w433]
      tunnel: [w349 w359 w381 w416 w431] -> w329
      tunnel: [w347 w355 w379 w415 OBJ_SCANNER_sequence_state."stop" ("state")] -> w326
      tunnel: [_ _ _ _ TRUE] -> w328
      tunnel: w327 -> [w344 w360 w372 w419 _]
      tunnel: [w333 w351 w377 w425 refnum<visa-resource-name> refnum ("VISA resource name out")] -> w325
      tunnel: w323 -> [_ w351 w377 w425 w430]
      tunnel: w322 -> [_ w357 w368 _ _]
      tunnel: ["" w357 w370 "" ""] -> w324
      frame "initialize" {
        n139 = Unbundle By Name(w344) -> ("main_ini_file.SCANNER Termination char"=w334:u8, "main_ini_file.SCANNER COM port"=w343:u16, "main_ini_file.SCANNER Baud rate"=w339:u32, "main_ini_file.SCANNER Data bits"=w338:u16, "main_ini_file.SCANNER Pairity"=w337:enum16{"None", "Odd", "Even", "Mark", "Space"}, "main_ini_file.SCANNER Stop bits"=w336:u16, "main_ini_file.SCANNER Flow control"=w335:u16)
        n140 = Number To Decimal String(number=w343) -> (decimal integer string=w342:string)  [unwired: 1 in]
        n141 = Concatenate Strings("COM" ("string"), w342) -> (w340:string)
        n142 = call-poly "VISA Configure Serial Port"("VISA resource name"=w340, "timeout (10sec)"=u32 150, "termination char\n(0xA = '\\n' = LF)"=w334, "baud rate (9600)"=w339, "data bits (8)"=w338, "parity (0:none)"=w337, "error in (no error)"=w346, "stop bits (10: 1 bit)"=w336, "flow control (0:none)"=w335) -> ("VISA resource name out"=w333:refnum<visa-resource-name>, "error out"=w345:errorcluster)  [unwired: 1 in, 4 out]
        n143 = call "OBJ_SCANNER_check_for_error.vi"("SCANNER_loop_state_in"=OBJ_SCANNER_sequence_state."get_next_state" ("SQL_EDITOR_sequence_state"), "error_in"=w345) -> ("SCANNER_loop_state_out"=w347:T9, "error_out"=w349:errorcluster)  [unwired: 8 in]
      }
      frame "get_next_state" {
        n144 = Unbundle By Name(w360) -> ("queue_refnums.SCANNER_queue"=w362:refnum<queue>)
        n145 = Dequeue Element(queue=w362, timeout in ms (-1)=0, error in (no error)=w361) -> (element=w350:T24, timed out?=w352:bool, error out=w354:errorcluster)  [unwired: 1 out]
        n146 = case shown="True" w352 {
          tunnel: w350 -> [w365 _]
          tunnel: [w363 OBJ_SCANNER_sequence_state."read" ("REWORK_SCANNER_sequence_state")] -> w356
          tunnel: [w364 w367] -> w353
          tunnel: w354 -> [w364 w367]
          frame False {
            n147 = Unbundle By Name(w365) -> ("state"=w363:T9)
          }
          frame True {
          }
        }
        n148 = call "OBJ_SCANNER_check_for_error.vi"("SCANNER_loop_state_in"=w356, "error_in"=w353) -> ("SCANNER_loop_state_out"=w355:T9, "error_out"=w359:errorcluster)  [unwired: 8 in]
      }
      frame "read" {
        # "timeout"
        n149 = VISA Read(VISA resource name=w377, byte count=u32 9999, error in (no error)=w378) -> (read buffer=w371:string, return count=w373:u32, error out=w369:errorcluster)  [unwired: 1 out]
        n150 = case shown="No Error" w369 {
          tunnel: w373 -> [_ w408]
          tunnel: w372 -> [w389 _]
          tunnel: w371 -> [w385 w407]
          tunnel: [w388 w406] -> w370
          tunnel: w368 -> [w386 w405]
          frame No Error {
            # "no (timeout) error means that termination character was encountered"
            n151 = Concatenate Strings(w386, w385) -> (w383:string)
            n152 = call <vilib>:"Trim Whitespace.vi"("string"=w383) -> ("trimmed string"=w382:string)  [unwired: 1 in]
            n153 = Not Equal?(x=w383, y="NoRead\r\n" ("x")) -> (x != y?=w384:bool)
            n154 = case shown="True" w384 {
              tunnel: w389 -> [w394 _]
              tunnel: ["" ""] -> w388
              tunnel: w382 -> [w390 _]
              frame True {
                # "read successful - send data and start new read"
                n155 = call "FGV_OBJ_login.vi"("options"=FGV_OBJ_login."get_login_info") -> ("Login read active?"=w391:bool)  [unwired: 6 in, 4 out]
                n156 = case shown="False" w391 {
                  tunnel: w394 -> [w397 w403]
                  tunnel: w390 -> [w395 w398]
                  frame True {
                    n157 = Unbundle By Name(w397) -> ("queue_refnums.SCANNER_login"=w396:refnum<queue>)
                    n158 = Lossy Enqueue Element(queue=w396, element=w395) -> ()  [unwired: 1 in, 4 out]
                  }
                  frame False {
                    n159 = Unbundle By Name(w403) -> ("queue_refnums.MAIN_queue"=w402:refnum<queue>)
                    n160 = To Variant(anything=w398) -> (Variant=w399:variant)
                    n161 = Bundle By Name(cluster=T23 {"state"=enum."read_gear_data", "variable"=variant} ("element"), "variable"=w399) -> (w400:T23)
                    n162 = Enqueue Element(queue=w402, element=w400) -> ()  [unwired: 2 in, 3 out]
                  }
                }
              }
              frame False {
                # "read completed, but unsuccessful - clear buffer and start read again"
              }
            }
          }
          frame Error {
            # "(timeout) error and some bytes read means that timeout occured before encountering termination character"
            n163 = case shown="0" w408 {
              tunnel: w407 -> [w410 _]
              tunnel: [w409 w412] -> w406
              tunnel: w405 -> [w411 w412]
              frame Default {
                # "if error and some bytes read, append new bytes (probably timeout, if not error case will take care of it)"
                n164 = Concatenate Strings(w411, w410) -> (w409:string)
              }
              frame 0 {
                # "if error and no bytes read, do nothing (probably timeout, if not error case will take care of it)"
                # "if error and no bytes read, do nothing (probably timeout, if not error case takes care of it"
              }
            }
          }
        }
        n165 = call <vilib>:"Clear Errors.vi"("error in (no error)"=w369, "specific error code to clear (0: all)"=-1073807339) -> ("error out"=w375:errorcluster)  [unwired: 4 in, 1 out]
        n166 = call "OBJ_SCANNER_check_for_error.vi"("SCANNER_loop_state_in"=OBJ_SCANNER_sequence_state."get_next_state" ("state"), "error_in"=w375) -> ("SCANNER_loop_state_out"=w379:T9, "error_out"=w381:errorcluster)  [unwired: 8 in]
      }
      frame "error" {
        n167 = Unbundle By Name(w419) -> ("queue_refnums.SCANNER_queue"=w418:refnum<queue>)
        n168 = call "FGV_OBJ_error_buffer.vi"("thread"=OBJ_thread."SCANNER", "option"=FGV_OBJ_error_buffer."display", "error_in"=w424) -> ("error_out"=w417:errorcluster)  [unwired: 7 in, 1 out]
        n169 = Preview Queue Element(queue=w418, timeout in ms (-1)=0, error in (no error)=w417) -> (element=w422:T24, error out=w416:errorcluster)  [unwired: 2 out]
        n170 = Unbundle By Name(w422) -> ("state"=w420:T9)
        n171 = case shown="Default" w420 {
          tunnel: [OBJ_SCANNER_sequence_state."initialize" ("state") OBJ_SCANNER_sequence_state."stop" ("state")] -> w415
          frame Default {
          }
          frame "stop" {
          }
        }
        n172 = call "wait_on_initialization.vi"("state"=w415) -> ()  [unwired: 11 in]
      }
      frame "stop" {
        # "1. takes so long to close it\nmaybe its not needed?\n2. works faster on server and is needed\nerrors after restart if not closed properly"
        n173 = call <vilib>:"Clear Errors.vi"("error in (no error)"=w433) -> ("error out"=w432:errorcluster)  [unwired: 5 in, 1 out]
        n174 = VISA Close(VISA resource name=w430, error in (no error)=w432) -> (error out=w431:errorcluster)
      }
    }
  }
  n175 = while {
    tunnel: w19 -> [w444]
    shift-right: [w441] -> _
    shift-left: "" -> [w440]
    shift-right: [w442] -> _
    shift-left: FALSE -> [w439]
    shift-right: [w443] -> _
    shift-left: _ -> [w438]
    shift-right: [w436] -> _
    shift-left: OBJ_MD_sequence_state."initialize" ("MD_loop_state_in") -> [w437]
    shift-right: [w445] -> w64
    shift-left: w17 -> [w446]
    stop <- w447 stop-if-true
    # "MEASURING DEVICE LEFT"
    n176 = case shown="\"initialize\"" w437 {
      tunnel: w446 -> [w465 w480 w502 w544 w554]
      tunnel: [w467 w478 w515 w535 w552] -> w445
      tunnel: [w466 w473 w513 w534 OBJ_MD_sequence_state."stop" ("state")] -> w436
      tunnel: [_ _ _ _ TRUE] -> w447
      tunnel: w444 -> [w463 w479 w508 w538 _]
      tunnel: [w452 w469 w501 w545 refnum<visa-resource-name> refnum ("VISA resource name out")] -> w443
      tunnel: w438 -> [_ w469 w501 w545 w551]
      tunnel: w439 -> [_ w477 _ _ _]
      tunnel: [FALSE w477 FALSE FALSE FALSE] -> w442
      tunnel: w440 -> [_ w475 w504 _ _]
      tunnel: ["" w475 w506 "" ""] -> w441
      frame "initialize" {
        n177 = Unbundle By Name(w463) -> ("main_ini_file.MD-L Termination char"=w453:u8, "main_ini_file.MD-L COM port"=w462:u16, "main_ini_file.MD-L Baud rate"=w458:u32, "main_ini_file.MD-L Data bits"=w457:u16, "main_ini_file.MD-L Pairity"=w456:enum16{"None", "Odd", "Even", "Mark", "Space"}, "main_ini_file.MD-L Stop bits"=w455:u16, "main_ini_file.MD-L Flow control"=w454:u16)
        n178 = Number To Decimal String(number=w462) -> (decimal integer string=w461:string)  [unwired: 1 in]
        n179 = Concatenate Strings("COM" ("string"), w461) -> (w459:string)
        n180 = call-poly "VISA Configure Serial Port"("VISA resource name"=w459, "timeout (10sec)"=u32 1000, "termination char\n(0xA = '\\n' = LF)"=w453, "baud rate (9600)"=w458, "data bits (8)"=w457, "parity (0:none)"=w456, "error in (no error)"=w465, "stop bits (10: 1 bit)"=w455, "flow control (0:none)"=w454) -> ("VISA resource name out"=w452:refnum<visa-resource-name>, "error out"=w464:errorcluster)  [unwired: 1 in, 4 out]
        n181 = call "OBJ_MD_check_for_error.vi"("MD_loop_state_in"=OBJ_MD_sequence_state."get_next_state", "error_in"=w464) -> ("MD_loop_state_out"=w466:T4, "error_out"=w467:errorcluster)  [unwired: 8 in]
      }
      frame "get_next_state" {
        n182 = case shown="False" w477 {
          tunnel: [-1 ("timeout in ms (-1)") 0 ("timeout in ms (-1)")] -> w476
          frame False {
          }
          frame True {
          }
        }
        n183 = Unbundle By Name(w479) -> ("queue_refnums.MD_L_queue"=w481:refnum<queue>)
        n184 = Dequeue Element(queue=w481, timeout in ms (-1)=w476, error in (no error)=w480) -> (element=w468:T25, timed out?=w470:bool, error out=w472:errorcluster)  [unwired: 1 out]
        n185 = case shown="False" w470 {
          tunnel: w468 -> [w482 _]
          tunnel: [w483 OBJ_MD_sequence_state."get_measurement" ("OBJ_MD_sequence_state")] -> w474
          tunnel: [w486 w495] -> w471
          tunnel: w472 -> [w487 w495]
          tunnel: w469 -> [w485 _]
          frame False {
            # "clear buffers\non read start"
            n186 = Unbundle By Name(w482) -> ("state"=w484:T4)
            n187 = case shown="Default" w484 {
              selector: w484 -> [w489 w490]
              tunnel: w487 -> [w488 w493]
              tunnel: [w488 w492] -> w486
              tunnel: w485 -> [_ w491]
              tunnel: [w489 w490] -> w483
              frame Default {
              }
              frame "get_measurement" {
                n188 = VISA Clear(VISA resource name=w491, error in (no error)=w493) -> (error out=w492:errorcluster)  [unwired: 1 out]
              }
            }
          }
          frame True {
          }
        }
        n189 = call "OBJ_MD_check_for_error.vi"("MD_loop_state_in"=w474, "error_in"=w471) -> ("MD_loop_state_out"=w473:T4, "error_out"=w478:errorcluster)  [unwired: 8 in]
      }
      frame "get_measurement" {
        # "experimental - only one read\nif working clean it up afterwards"
        # "timeout"
        n190 = VISA Write(VISA resource name=w501, write buffer="1\r\n", error in (no error)=w502) -> (VISA resource name out=w500:refnum<visa-resource-name>, error out=w503:errorcluster)  [unwired: 1 out]
        n191 = VISA Read(VISA resource name=w500, byte count=u32 9999, error in (no error)=w503) -> (read buffer=w507:string, return count=w509:u32, error out=w505:errorcluster)  [unwired: 1 out]
        n192 = case shown="Error .." w505 {
          tunnel: w509 -> [_ w527]
          tunnel: w508 -> [w522 w526]
          tunnel: w507 -> [w519 w525]
          tunnel: ["" w524] -> w506
          tunnel: w504 -> [w520 w523]
          frame No Error {
            # "no (timeout) error means that read was performed"
            n193 = Concatenate Strings(w520, w519) -> (w518:string)
            n194 = call <vilib>:"Trim Whitespace.vi"("string"=w518) -> ("trimmed string"=w516:string)  [unwired: 1 in]
            n195 = Unbundle By Name(w522) -> ("queue_refnums.MD_L_data"=w517:refnum<queue>)
            n196 = Lossy Enqueue Element(queue=w517, element=w516) -> ()  [unwired: 1 in, 4 out]
          }
          frame Error {
            # "(timeout) error and some bytes read means that timeout occured before encountering termination character"
            n197 = case shown="0" w527 {
              tunnel: w526 -> [_ _]
              tunnel: w525 -> [w529 _]
              tunnel: [w528 w531] -> w524
              tunnel: w523 -> [w530 w531]
              frame Default {
                # "if error and some bytes read, append new bytes (probably timeout, if not error case will take care of it)"
                n198 = Concatenate Strings(w530, w529) -> (w528:string)
              }
              frame 0 {
                # "if error and no bytes read, do nothing (probably timeout, if not error case will take care of it)"
                # "if error and no bytes read, do nothing (probably timeout, if not error case takes care of it"
              }
            }
          }
        }
        n199 = call <vilib>:"Clear Errors.vi"("error in (no error)"=w505, "specific error code to clear (0: all)"=-1073807339) -> ("error out"=w511:errorcluster)  [unwired: 4 in, 1 out]
        n200 = call "OBJ_MD_check_for_error.vi"("MD_loop_state_in"=OBJ_MD_sequence_state."get_next_state" ("state"), "error_in"=w511) -> ("MD_loop_state_out"=w513:T4, "error_out"=w515:errorcluster)  [unwired: 8 in]
      }
      frame "error" {
        n201 = Unbundle By Name(w538) -> ("queue_refnums.MD_L_queue"=w537:refnum<queue>)
        n202 = call "FGV_OBJ_error_buffer.vi"("thread"=OBJ_thread."MD - LEFT", "option"=FGV_OBJ_error_buffer."display", "error_in"=w544) -> ("error_out"=w536:errorcluster)  [unwired: 7 in, 1 out]
        n203 = Preview Queue Element(queue=w537, timeout in ms (-1)=0, error in (no error)=w536) -> (element=w541:T25, error out=w535:errorcluster)  [unwired: 2 out]
        n204 = Unbundle By Name(w541) -> ("state"=w539:T4)
        n205 = case shown="\"stop\"" w539 {
          tunnel: [OBJ_MD_sequence_state."initialize" ("state") OBJ_MD_sequence_state."stop" ("state")] -> w534
          frame Default {
          }
          frame "stop" {
          }
        }
        n206 = call "wait_on_initialization.vi"("state"=w534) -> ()  [unwired: 11 in]
      }
      frame "stop" {
        # "1. takes so long to close it\nmaybe its not needed?\n2. works faster on server and is needed\nerrors after restart if not closed properly"
        n207 = call <vilib>:"Clear Errors.vi"("error in (no error)"=w554) -> ("error out"=w553:errorcluster)  [unwired: 5 in, 1 out]
        n208 = VISA Close(VISA resource name=w551, error in (no error)=w553) -> (error out=w552:errorcluster)
      }
    }
  }
  n209 = while {
    tunnel: w19 -> [w565]
    shift-right: [w562] -> _
    shift-left: "" -> [w559]
    shift-right: [w563] -> _
    shift-left: FALSE -> [w560]
    shift-right: [w564] -> _
    shift-left: _ -> [w561]
    shift-right: [w557] -> _
    shift-left: OBJ_MD_sequence_state."initialize" ("MD_loop_state_in") -> [w558]
    shift-right: [w567] -> w63
    shift-left: w17 -> [w566]
    stop <- w568 stop-if-true
    # "MEASURING DEVICE RIGHT"
    n210 = case shown="\"initialize\"" w558 {
      tunnel: w566 -> [w586 w601 w623 w665 w675]
      tunnel: [w588 w599 w636 w656 w673] -> w567
      tunnel: [w587 w594 w634 w655 OBJ_MD_sequence_state."stop" ("state")] -> w557
      tunnel: [_ _ _ _ TRUE] -> w568
      tunnel: w565 -> [w584 w600 w629 w659 _]
      tunnel: [w573 w590 w622 w666 refnum<visa-resource-name> refnum ("VISA resource name out")] -> w564
      tunnel: w561 -> [_ w590 w622 w666 w672]
      tunnel: w560 -> [_ w598 _ _ _]
      tunnel: [FALSE w598 FALSE FALSE FALSE] -> w563
      tunnel: w559 -> [_ w596 w625 _ _]
      tunnel: ["" w596 w627 "" ""] -> w562
      frame "initialize" {
        n211 = Unbundle By Name(w584) -> ("main_ini_file.MD-R Termination char"=w574:u8, "main_ini_file.MD-R COM port"=w583:u16, "main_ini_file.MD-R Baud rate"=w579:u32, "main_ini_file.MD-R Data bits"=w578:u16, "main_ini_file.MD-R Pairity"=w577:enum16{"None", "Odd", "Even", "Mark", "Space"}, "main_ini_file.MD-R Stop bits"=w576:u16, "main_ini_file.MD-R Flow control"=w575:u16)
        n212 = Number To Decimal String(number=w583) -> (decimal integer string=w582:string)  [unwired: 1 in]
        n213 = Concatenate Strings("COM" ("string"), w582) -> (w580:string)
        n214 = call-poly "VISA Configure Serial Port"("VISA resource name"=w580, "timeout (10sec)"=u32 1000, "termination char\n(0xA = '\\n' = LF)"=w574, "baud rate (9600)"=w579, "data bits (8)"=w578, "parity (0:none)"=w577, "error in (no error)"=w586, "stop bits (10: 1 bit)"=w576, "flow control (0:none)"=w575) -> ("VISA resource name out"=w573:refnum<visa-resource-name>, "error out"=w585:errorcluster)  [unwired: 1 in, 4 out]
        n215 = call "OBJ_MD_check_for_error.vi"("MD_loop_state_in"=OBJ_MD_sequence_state."get_next_state", "error_in"=w585) -> ("MD_loop_state_out"=w587:T4, "error_out"=w588:errorcluster)  [unwired: 8 in]
      }
      frame "get_next_state" {
        n216 = case shown="False" w598 {
          tunnel: [-1 ("timeout in ms (-1)") 0 ("timeout in ms (-1)")] -> w597
          frame False {
          }
          frame True {
          }
        }
        n217 = Unbundle By Name(w600) -> ("queue_refnums.MD_R_queue"=w602:refnum<queue>)
        n218 = Dequeue Element(queue=w602, timeout in ms (-1)=w597, error in (no error)=w601) -> (element=w589:T25, timed out?=w591:bool, error out=w593:errorcluster)  [unwired: 1 out]
        n219 = case shown="False" w591 {
          tunnel: w589 -> [w603 _]
          tunnel: [w604 OBJ_MD_sequence_state."get_measurement" ("OBJ_MD_sequence_state")] -> w595
          tunnel: [w607 w616] -> w592
          tunnel: w593 -> [w608 w616]
          tunnel: w590 -> [w606 _]
          frame False {
            # "clear buffers\non read start"
            n220 = Unbundle By Name(w603) -> ("state"=w605:T4)
            n221 = case shown="Default" w605 {
              selector: w605 -> [w610 w611]
              tunnel: w608 -> [w609 w614]
              tunnel: [w609 w613] -> w607
              tunnel: w606 -> [_ w612]
              tunnel: [w610 w611] -> w604
              frame Default {
              }
              frame "get_measurement" {
                n222 = VISA Clear(VISA resource name=w612, error in (no error)=w614) -> (error out=w613:errorcluster)  [unwired: 1 out]
              }
            }
          }
          frame True {
          }
        }
        n223 = call "OBJ_MD_check_for_error.vi"("MD_loop_state_in"=w595, "error_in"=w592) -> ("MD_loop_state_out"=w594:T4, "error_out"=w599:errorcluster)  [unwired: 8 in]
      }
      frame "get_measurement" {
        # "experimental - only one read\nif working clean it up afterwards"
        # "timeout"
        n224 = VISA Write(VISA resource name=w622, write buffer="1\r\n", error in (no error)=w623) -> (VISA resource name out=w621:refnum<visa-resource-name>, error out=w624:errorcluster)  [unwired: 1 out]
        n225 = VISA Read(VISA resource name=w621, byte count=u32 9999, error in (no error)=w624) -> (read buffer=w628:string, return count=w630:u32, error out=w626:errorcluster)  [unwired: 1 out]
        n226 = case shown="Error .." w626 {
          tunnel: w630 -> [_ w648]
          tunnel: w629 -> [w643 w647]
          tunnel: w628 -> [w640 w646]
          tunnel: ["" w645] -> w627
          tunnel: w625 -> [w641 w644]
          frame No Error {
            # "no (timeout) error means that read was performed"
            n227 = Concatenate Strings(w641, w640) -> (w639:string)
            n228 = call <vilib>:"Trim Whitespace.vi"("string"=w639) -> ("trimmed string"=w637:string)  [unwired: 1 in]
            n229 = Unbundle By Name(w643) -> ("queue_refnums.MD_R_data"=w638:refnum<queue>)
            n230 = Lossy Enqueue Element(queue=w638, element=w637) -> ()  [unwired: 1 in, 4 out]
          }
          frame Error {
            # "(timeout) error and some bytes read means that timeout occured before encountering termination character"
            n231 = case shown="0" w648 {
              tunnel: w647 -> [_ _]
              tunnel: w646 -> [w650 _]
              tunnel: [w649 w652] -> w645
              tunnel: w644 -> [w651 w652]
              frame Default {
                # "if error and some bytes read, append new bytes (probably timeout, if not error case will take care of it)"
                n232 = Concatenate Strings(w651, w650) -> (w649:string)
              }
              frame 0 {
                # "if error and no bytes read, do nothing (probably timeout, if not error case will take care of it)"
                # "if error and no bytes read, do nothing (probably timeout, if not error case takes care of it"
              }
            }
          }
        }
        n233 = call <vilib>:"Clear Errors.vi"("error in (no error)"=w626, "specific error code to clear (0: all)"=-1073807339) -> ("error out"=w632:errorcluster)  [unwired: 4 in, 1 out]
        n234 = call "OBJ_MD_check_for_error.vi"("MD_loop_state_in"=OBJ_MD_sequence_state."get_next_state" ("state"), "error_in"=w632) -> ("MD_loop_state_out"=w634:T4, "error_out"=w636:errorcluster)  [unwired: 8 in]
      }
      frame "error" {
        n235 = Unbundle By Name(w659) -> ("queue_refnums.MD_R_queue"=w658:refnum<queue>)
        n236 = call "FGV_OBJ_error_buffer.vi"("thread"=OBJ_thread."MD - RIGHT", "option"=FGV_OBJ_error_buffer."display", "error_in"=w665) -> ("error_out"=w657:errorcluster)  [unwired: 7 in, 1 out]
        n237 = Preview Queue Element(queue=w658, timeout in ms (-1)=0, error in (no error)=w657) -> (element=w662:T25, error out=w656:errorcluster)  [unwired: 2 out]
        n238 = Unbundle By Name(w662) -> ("state"=w660:T4)
        n239 = case shown="\"stop\"" w660 {
          tunnel: [OBJ_MD_sequence_state."initialize" ("state") OBJ_MD_sequence_state."stop" ("state")] -> w655
          frame Default {
          }
          frame "stop" {
          }
        }
        n240 = call "wait_on_initialization.vi"("state"=w655) -> ()  [unwired: 11 in]
      }
      frame "stop" {
        # "1. takes so long to close it\nmaybe its not needed?\n2. works faster on server and is needed\nerrors after restart if not closed properly"
        n241 = call <vilib>:"Clear Errors.vi"("error in (no error)"=w675) -> ("error out"=w674:errorcluster)  [unwired: 5 in, 1 out]
        n242 = VISA Close(VISA resource name=w672, error in (no error)=w674) -> (error out=w673:errorcluster)
      }
    }
  }
  n243 = while {
    tunnel: w19 -> [w685]
    shift-right: [w682] -> _
    shift-left: OBJ_GUI_TIMER_sequence_state."initialize" ("OBJ_GUI_TIMER_sequence_state") -> [w684]
    shift-right: [w681] -> w15
    shift-left: w17 -> [w683]
    shift-right: [w680] -> _
    shift-left: FALSE -> [w679]
    stop <- w678 stop-if-true
    # "GUI CLEAR TIMER"
    n244 = case shown="\"initialize\"" w684 {
      tunnel: w685 -> [_ w703 _ _ _ w731 _]
      tunnel: w683 -> [w690 w702 w710 w715 w721 w730 w741]
      tunnel: [w688 w695 w712 w717 w724 w728 OBJ_GUI_TIMER_sequence_state."stop" ("OBJ_GUI_TIMER_sequence_state")] -> w682
      tunnel: [w689 w696 w713 w718 w725 w729 w741] -> w681
      tunnel: [FALSE w701 TRUE FALSE FALSE FALSE FALSE] -> w680
      tunnel: w679 -> [_ w701 _ _ _ _ _]
      tunnel: [_ _ _ _ _ _ TRUE] -> w678
      frame "initialize" {
        n245 = call "OBJ_GUI_TIMER_check_for_error.vi"("GUI_TIMER_loop_state_in"=OBJ_GUI_TIMER_sequence_state."get_next_state", "error_in"=w690) -> ("GUI_TIMER_loop_state_out"=w688:T2, "error_out"=w689:errorcluster)  [unwired: 8 in]
      }
      frame "get_next_state" {
        n246 = Unbundle By Name(w703) -> ("queue_refnums.OBJ_GUI_TIMER_queue"=w704:refnum<queue>)
        n247 = Select(t=10000, s=w701, f=-1 ("timeout in ms (-1)")) -> (s? t:f=w698:i32)
        n248 = Dequeue Element(queue=w704, timeout in ms (-1)=w698, error in (no error)=w702) -> (element=w693:T21, timed out?=w697:bool, error out=w694:errorcluster)  [unwired: 1 out]
        n249 = case shown="True" w697 {
          tunnel: w694 -> [w707 w709]
          tunnel: w693 -> [w706 _]
          tunnel: [w707 w709] -> w692
          tunnel: [w705 OBJ_GUI_TIMER_sequence_state."timer_finished" ("state")] -> w691
          frame False {
            n250 = Unbundle By Name(w706) -> ("state"=w705:T2)
          }
          frame True {
          }
        }
        n251 = call "OBJ_GUI_TIMER_check_for_error.vi"("GUI_TIMER_loop_state_in"=w691, "error_in"=w692) -> ("GUI_TIMER_loop_state_out"=w695:T2, "error_out"=w696:errorcluster)  [unwired: 8 in]
      }
      frame "start_timer" {
        n252 = call "OBJ_GUI_TIMER_check_for_error.vi"("GUI_TIMER_loop_state_in"=OBJ_GUI_TIMER_sequence_state."get_next_state", "error_in"=w710) -> ("GUI_TIMER_loop_state_out"=w712:T2, "error_out"=w713:errorcluster)  [unwired: 8 in]
      }
      frame "stop_timer" {
        n253 = call "OBJ_GUI_TIMER_check_for_error.vi"("GUI_TIMER_loop_state_in"=OBJ_GUI_TIMER_sequence_state."get_next_state", "error_in"=w715) -> ("GUI_TIMER_loop_state_out"=w717:T2, "error_out"=w718:errorcluster)  [unwired: 8 in]
      }
      frame "timer_finished" {
        n254 = call "FGV_tristate_indicator_OBJ_test.vi"("options"=FGV_tristate_indicator_OBJ_test."timeout", "error_in"=w721) -> ("error_out"=w720:errorcluster)  [unwired: 9 in]
        n255 = call "OBJ_GUI_TIMER_check_for_error.vi"("GUI_TIMER_loop_state_in"=OBJ_GUI_TIMER_sequence_state."get_next_state", "error_in"=w720) -> ("GUI_TIMER_loop_state_out"=w724:T2, "error_out"=w725:errorcluster)  [unwired: 8 in]
      }
      frame "error" {
        n256 = Unbundle By Name(w731) -> ("queue_refnums.OBJ_GUI_TIMER_queue"=w737:refnum<queue>)
        n257 = call "FGV_OBJ_error_buffer.vi"("thread"=OBJ_thread."GUI TIMER", "option"=FGV_OBJ_error_buffer."display", "error_in"=w730) -> ("error_out"=w738:errorcluster)  [unwired: 7 in, 1 out]
        n258 = Preview Queue Element(queue=w737, timeout in ms (-1)=0, error in (no error)=w738) -> (element=w735:T21, error out=w729:errorcluster)  [unwired: 2 out]
        n259 = Unbundle By Name(w735) -> ("state"=w736:T2)
        n260 = case shown="\"stop\"" w736 {
          tunnel: [OBJ_GUI_TIMER_sequence_state."initialize" ("OBJ_GUI_TIMER_sequence_state") OBJ_GUI_TIMER_sequence_state."stop" ("OBJ_GUI_TIMER_sequence_state")] -> w728
          frame Default {
          }
          frame "stop" {
          }
        }
        n261 = call "wait_on_initialization.vi"("state"=w728) -> ()  [unwired: 11 in]
      }
      frame "stop" {
      }
    }
  }
  n262 = while {
    tunnel: w17 -> [w747]
    tunnel: [w749] -> w69
    tunnel: w19 -> [w746]
    tunnel: w21 -> [w745]
    stop <- w748 stop-if-true
    # "EVENTS"
    n263 = event shown="[1] \"USER_login_logout\": Value Change" {
      selector: _ -> [_ _ _ _ _ _ _ _ _ _ _]
      dyn-events: _ -> [_ _ _ _ _ _ _ _ _ _ _]
      timeout: w745 -> [_ _ _ _ _ _ _ _ _ _ _]
      tunnel: w747 -> [w757 w763 w790 w794 w797 w801 w806 w818 w821 w844 w849]
      tunnel: [w756 w759 w790 w794 w796 w800 w805 w818 w821 w844 w852] -> w749
      tunnel: [_ _ _ _ _ _ _ _ _ _ w851] -> w748
      tunnel: w746 -> [w755 w765 _ _ w795 _ w804 _ _ _ w847]
      event "OBJ_perform_test": Value Change {
        n264 = event-data() -> ()  [unwired: 1 in, 6 out]
        n265 = local read "OBJ_gear_serial"() -> (w750:string)
        n266 = Unbundle By Name(w755) -> ("queue_refnums.MAIN_queue"=w754:refnum<queue>)
        n267 = To Variant(anything=w750) -> (Variant=w751:variant)
        n268 = Bundle By Name(cluster=T23 {"state"=enum."read_gear_data", "variable"=variant} ("element"), "variable"=w751) -> (w752:T23)
        n269 = Enqueue Element(queue=w754, element=w752, error in (no error)=w757) -> (error out=w756:errorcluster)  [unwired: 1 in, 2 out]
      }
      event "USER_login_logout": Value Change {
        n270 = event-data() -> ()  [unwired: 1 in, 6 out]
        n271 = call "FGV_OBJ_login.vi"("options"=FGV_OBJ_login."start_login_read", "error_in"=w763) -> ("error_out"=w762:errorcluster)  [unwired: 5 in, 4 out]
        n272 = local read "current_access_level"() -> (w764:i32)
        n273 = case shown="0" w764 {
          tunnel: [w771 w785] -> w760
          tunnel: w762 -> [w770 w783]
          tunnel: w765 -> [w766 w782]
          frame 0 {
            n274 = call "OBJ_LOGIN_scan_barcode.vi"("error_in"=w770, "all_config_info"=w766) -> ("error_out"=w769:errorcluster, "Canceled?"=w767:bool, "barcode"=w768:string)  [unwired: 7 in]
            n275 = case shown="False" w767 {
              tunnel: [w779 w780] -> w771
              tunnel: w769 -> [w776 w780]
              tunnel: w766 -> [w775 _]
              tunnel: w768 -> [w774 _]
              frame False {
                n276 = Unbundle By Name(w775) -> ("queue_refnums.MAIN_queue"=w778:refnum<queue>)
                n277 = To Variant(anything=w774) -> (Variant=w777:variant)
                n278 = Bundle By Name(cluster=T23 {"state"=enum."USER_login", "variable"=variant} ("element"), "variable"=w777) -> (w772:T23)
                n279 = Enqueue Element(queue=w778, element=w772, error in (no error)=w776) -> (error out=w779:errorcluster)  [unwired: 1 in, 2 out]
              }
              frame True {
              }
            }
          }
          frame Default {
            n280 = Unbundle By Name(w782) -> ("queue_refnums.MAIN_queue"=w784:refnum<queue>)
            n281 = Enqueue Element(queue=w784, element=T23 {"state"=enum."USER_logout", "variable"=variant}, error in (no error)=w783) -> (error out=w785:errorcluster)  [unwired: 1 in, 2 out]
          }
        }
        n282 = call "FGV_OBJ_login.vi"("options"=FGV_OBJ_login."end_login_read", "error_in"=w760) -> ("error_out"=w759:errorcluster)  [unwired: 5 in, 4 out]
      }
      event "current_access_level": Value Change {
        n283 = event-data() -> ("NewVal"=w789:i32)  [unwired: 1 in]
        n284 = case shown="1..10" w789 {
          tunnel: [w791 w792] -> w786
          frame Default {
            w791 = enum32{"OBJ Test", "Errors"}[] [enum."Errors"] items=["OBJ Test", "Errors"]
          }
          frame 1..10 {
            w792 = enum32{"OBJ Test", "Errors"}[] [enum."OBJ Test", enum."Errors"] items=["OBJ Test", "Errors"]
          }
        }
        n285 = control-ref of="main_tab"() -> (w787:refnum<vi>)
        n286 = control-ref of="This VI"() -> (w788:refnum<vi>)
        n287 = call "OBJ_show_hide_pages.vi"("This VI"=w788, "visible_pages"=w786, "main_tab_ref"=w787) -> ()  [unwired: 9 in]
      }
      event "ERROR_clear": Value Change {
        n288 = event-data() -> ()  [unwired: 1 in, 6 out]
        n289 = call "FGV_OBJ_error_buffer.vi"("option"=FGV_OBJ_error_buffer."clear") -> ()  [unwired: 9 in, 2 out]
      }
      event "OBJ_clear_test_data": Value Change {
        n290 = event-data() -> ()  [unwired: 1 in, 6 out]
        n291 = Unbundle By Name(w795) -> ("queue_refnums.MAIN_queue"=w799:refnum<queue>)
        n292 = Enqueue Element(queue=w799, element=T23 {"state"=enum."clear_test_data", "variable"=variant}, error in (no error)=w797) -> (error out=w796:errorcluster)  [unwired: 1 in, 2 out]
      }
      event "OBJ_clear_history": Value Change {
        n293 = event-data() -> ()  [unwired: 1 in, 6 out]
        n294 = call "FGV_OBJ_history_display.vi"("options"=FGV_OBJ_history_display."clear", "error_in"=w801) -> ("error_out"=w800:errorcluster)  [unwired: 9 in]
      }
      event Timeout {
        n295 = event-data() -> ()  [unwired: 1 in, 3 out]
        n296 = Unbundle By Name(w804) -> ("queue_refnums.MAIN_queue"=w803:refnum<queue>)
        n297 = local read "current_access_level"() -> (w807:i32)
        n298 = case shown="Default" w807 {
          tunnel: w806 -> [w808 w812]
          tunnel: [w808 w816] -> w805
          tunnel: w803 -> [_ w810]
          frame 0 {
          }
          frame Default {
            n299 = Enqueue Element(queue=w810, element=T23 {"state"=enum."USER_logout", "variable"=variant}, error in (no error)=w812) -> (error out=w811:errorcluster)  [unwired: 1 in, 2 out]
            n300 = call "message_popup.vi"("Warning(T)/Info(F)"=TRUE, "error_in"=w811, "Message"="Automatic user logout was performed due to inactivity", "Title"="Automatic Logout", "Button Label"="OK") -> ("error_out"=w816:errorcluster)  [unwired: 6 in]
          }
        }
      }
      event "professional_timeout_reset_generator": Value Change {
        n301 = event-data() -> ()  [unwired: 1 in, 6 out]
      }
      event Menu Selection (User) {
        n302 = event-data() -> ("ItemTag"=w820:string)  [unwired: 1 in, 6 out]
        n303 = call "Get Key For Phrase.vi"("Phrase"=w820) -> ("Key"=w819:string)  [unwired: 9 in, 1 out]
        n304 = case shown="\"Language - English\", \"Language - Russian\"" w819 {
          selector: w819 -> [_ w828 _ _]
          frame Default {
          }
          frame "Language - English", "Language - Russian" {
            n305 = case shown="\"Language - Russian\"" w828 {
              tunnel: ["Russian" ("Target Language (current lang)") "English" ("Target Language (current lang)")] -> w829
              frame "Language - Russian" {
              }
              frame "Language - English", Default {
              }
            }
            n306 = call "Set Language.vi"("Target Language (current lang)"=w829) -> ("error out"=w827:errorcluster)  [unwired: 9 in, 1 out]
            n307 = Current VI's Menubar() -> (w826:refnum<k9>)
            n308 = call "OBJ_create_menu_bar.vi"("error_in"=w827, "menu_bar_refnum"=w826) -> ("error_out"=w825:errorcluster)  [unwired: 9 in]
            n309 = call "FGV_tristate_indicator_OBJ_test.vi"("options"=FGV_tristate_indicator_OBJ_test."translate", "error_in"=w825) -> ("error_out"=w822:errorcluster)  [unwired: 9 in]
            n310 = call "FGV_OBJ_test_button.vi"("options"=FGV_OBJ_test_button."translate", "error_in"=w822) -> ()  [unwired: 8 in, 2 out]
          }
          frame "About" {
            n311 = disable-structure shown="Default" {
              disable-tunnel: [w838 w841] -> w834
              disable-tunnel: [w839 w841] -> w833
              frame condition #0 {
                n312 = vi-ref "get_exe_compilation_date.vi"() -> (w840:refnum<vi>)
                n313 = call-by-ref "?"(reference=w840) -> ("compilation_time"=w838:string, "compilation_date"=w839:string)  [unwired: 10 in, 3 out]
              }
              frame condition #1 (active) {
                n314 = call-poly "Get Localized Phrase Compact Interface.vi"("Key"="NOT COMPILED!" ("compilation_date")) -> ("Translated Phrase"=w841:string)
              }
            }
            n315 = call-poly "Get Localized Phrase Compact Interface.vi"("Key"="SQL Proxy Application\nMSG Assembly Line\nA603A00\n\nAumatic sp. z o.o.\nPilsudskiego 22\n32-050 Skawina\nPOLAND\n\nCOMPILATION DATE: %s\nCOMPILATION TIME: %s\nJakub Longa, 2020\n\n+48 (12) 256-77-90\naumatic.com" ("about_string")) -> ("Translated Phrase"=w832:string)
            n316 = Format Into String(format string=w832, w833, w834) -> (resulting string=w837:string)  [unwired: 2 in, 1 out]
            n317 = call "about_window.vi"("lines_to_bold"=i32[] [0, 1, 4, 9], "about_string"=w837) -> ()  [unwired: 9 in, 1 out]
          }
          frame "Exit" {
            n318 = property on="STOP" class="Bool (strict)"("Val(Sgnl)"=TRUE ("Value (Signaling)")) -> ()  [unwired: 2 in, 2 out]
          }
        }
      }
      event Panel Close? {
        n319 = event-data() -> ()  [unwired: 1 in, 4 out]
        n320 = property on="STOP" class="Bool (strict)"("Val(Sgnl)"=TRUE ("Value (Signaling)")) -> ()  [unwired: 2 in, 2 out]
        n321 = event-data("Discard?"=TRUE) -> ()  [unwired: 1 in, 1 out]
      }
      event "STOP": Value Change {
        n322 = event-data() -> ()  [unwired: 1 in, 6 out]
        n323 = disable-structure shown="RUN_TIME_ENGINE==True" {
          disable-tunnel: [w855 TRUE ("Result")] -> w850
          disable-tunnel: w849 -> [w854 w866]
          disable-tunnel: [w853 w866] -> w848
          frame condition #0 {
            n324 = case shown="No Error" w854 {
              selector: w854 -> [w860 w863]
              tunnel: [w861 TRUE ("Result")] -> w855
              tunnel: [w859 w863] -> w853
              frame No Error {
                n325 = call "confirm_popup.vi"("Warning(T)/Inf(F)"=TRUE, "error_in"=w860, "False Label"="No", "True Label"="Yes", "Message"="Are you sure you want to exit the application?") -> ("error_out"=w859:errorcluster, "Result"=w861:bool)  [unwired: 5 in]
              }
              frame Error {
              }
            }
          }
          frame condition #1 (active) {
          }
        }
        n326 = case shown="True" w850 {
          tunnel: w848 -> [w867 w883]
          tunnel: [w867 w871] -> w852
          tunnel: [FALSE TRUE] -> w851
          tunnel: w847 -> [_ w882]
          frame False {
          }
          frame True {
            n327 = Unbundle By Name(w882) -> ("queue_refnums.OBJ_GUI_TIMER_queue"=w870:refnum<queue>, "queue_refnums.MAIN_queue"=w886:refnum<queue>, "queue_refnums.SCANNER_queue"=w884:refnum<queue>, "queue_refnums.MD_L_queue"=w878:refnum<queue>, "queue_refnums.MD_R_queue"=w877:refnum<queue>)
            n328 = call <vilib>:"Clear Errors.vi"("error in (no error)"=w883) -> ("error out"=w881:errorcluster)  [unwired: 5 in, 1 out]
            n329 = Enqueue Element At Opposite End(queue=w877, element=T25 {"state"=enum."stop", "variable"=variant}, error in (no error)=w881) -> (error out=w880:errorcluster)  [unwired: 1 in, 2 out]
            n330 = Enqueue Element At Opposite End(queue=w878, element=T25 {"state"=enum."stop", "variable"=variant}, error in (no error)=w880) -> (error out=w879:errorcluster)  [unwired: 1 in, 2 out]
            n331 = Enqueue Element At Opposite End(queue=w884, element=T24 {"state"=enum."stop", "variable"=variant}, error in (no error)=w879) -> (error out=w885:errorcluster)  [unwired: 1 in, 2 out]
            n332 = Enqueue Element At Opposite End(queue=w886, element=T23 {"state"=enum."stop", "variable"=variant}, error in (no error)=w885) -> (error out=w872:errorcluster)  [unwired: 1 in, 2 out]
            n333 = Enqueue Element At Opposite End(queue=w870, element=T21 {"state"=enum."stop", "variable"=variant}, error in (no error)=w872) -> (error out=w871:errorcluster)  [unwired: 1 in, 2 out]
          }
        }
      }
    }
  }
  n334 = Merge Errors(w15, w69, w66, w65, w64, w63) -> (w67:errorcluster)
  n335 = call "OBJ_destroy_queues.vi"("error_in"=w67, "all_config_info"=w19) -> ("error_out"=w68:errorcluster)  [unwired: 9 in]
  n336 = control-ref of="This VI"() -> (w71:refnum<vi>)
  n337 = call "close_front_panel_in_exe.vi"("error_in"=w68, "vi_reference_in"=w71) -> ("error_out"=w70:errorcluster)  [unwired: 9 in]
  n338 = call <vilib>:"Clear Errors.vi"("error in (no error)"=w70) -> ()  [unwired: 5 in, 2 out]
